vi "main.vi"() -> ()   [LabVIEW 2018]
uses:
  <vilib>/Platform/TimedLoop/XDataNode/timing_clust.ctl
  <vilib>/Platform/TimedLoop/XDataNode/nitl_modes.ctl
  <vilib>/Platform/TimedLoop/XDataNode/wakeup.ctl
  a5fe1e67-a595-4ba8-95b3-b389166d0479.vi
  fafd1210-cecf-4ec7-9a0a-c581520fbfe6.vi
  42531a82-c600-4602-b648-2c62e518af83.vi
  <vilib>/express/express shared/transition.llb/Dynamic To Waveform Array.vi
  <vilib>/express/express signal manip/GetorSetDDTAttributes/Set DDT Attributes/SetT0.vi
  <vilib>/express/express signal manip/GetorSetDDTAttributes/Set DDT Attributes/sub Set StartTimeStamp.vi
  <vilib>/express/express shared/transition.llb/Waveform Array To Dynamic.vi
  <vilib>/platform/TimedLoop/XDataNode/XDataNode.xnode
  <vilib>/express/express signal manip/GetorSetDDTAttributes/Set DDT Attributes/Set DDT Properties.xnode
  <vilib>/Platform/TimedLoop/XDataNode/XDNodeRunTimeDep.lvlib
  <vilib>/express/express signal manip/GetorSetDDTAttributes/Set DDT Attributes/Set DDT Attributes.lvlib
panel:
  in  "New file":bool
  out "Pending":i32
  out "RecordStatus":bool
  out "System State":T1(ring)
  in  "Overdrive":bool
  in  "Pause DAQ":bool
  in  "Record":bool
  in  "Log Folder":path=path "C:/LPLDocs"
  in  "Sensor Log Name":string="Log_Sensors"
  in  "Load Cell Log Name":string="Log_LoadCell"
  in  "Valve Log Name":string="Log_Valves"
  in  "Fire Sequence Tabs":T2(tab)
  in  "NC-F\nTiming":cluster{dbl, dbl, dbl, dbl, dbl, dbl}(slide)={0.0, 8.07, 10.0, 13.0, 13.0, 13.012830257415771} scale=0.0..13.0
  in  "NC-O\nTiming":cluster{dbl, dbl, dbl, dbl, dbl, dbl}(slide)={0.0, 8.05, 9.3, 13.0, 13.0, 13.012830257415771} scale=0.0..13.0
  in  "Ignitor\nTiming":cluster{dbl, dbl, dbl, dbl, dbl, dbl}(slide)={0.0, 9.8, 9.8, 13.0, 13.0, 13.012830257415771} scale=0.0..13.0
  in  "NC-FI\nTiming":cluster{dbl, dbl, dbl, dbl, dbl, dbl}(slide)={0.0, 15.0, 15.0, 15.0, 15.0, 0.0} scale=0.0..13.0
  in  "NC-OI\nTiming":cluster{dbl, dbl, dbl, dbl, dbl, dbl}(slide)={0.0, 15.0, 15.0, 15.0, 15.0, 0.0} scale=0.0..13.0
  in  "Fire\nTiming":cluster{dbl, dbl, dbl}(slide)={0.0, 10.0, 0.0} scale=0.0..13.0
  in  "NC-F Invert":bool
  in  "NC-O Invert":bool
  in  "Ignitor Invert":bool
  in  "NC-FI Invert":bool
  in  "NC-OI Invert":bool
  in  "ABORTED\nState":bool[](array[boolean])=[TRUE, TRUE, FALSE, FALSE, FALSE, FALSE]
  out "ABORTED Indicator":bool
  in  "Ignition Type":u16(ring)=2 items=["Spark Plug", "Glow Plug", "Pyrotechnic"]
  in  "Countdown + Fring\nLength":dbl=13.0
  in  "NC-F Open Delay":dbl=1.93
  in  "NC-O Open Delay":dbl=1.25
  in  "NC-FI Open Delay":dbl
  in  "Igniter Active Delay":dbl=1.0
  in  "NC-OI Open Delay":dbl
  in  "NC-F Close Delay":dbl
  in  "NC-O Close Delay":dbl
  in  "NC-FI Close Delay":dbl
  in  "Igniter Inactive Delay":dbl
  in  "NC-OI Close Delay":dbl
  in  "Edit Fire \nSequence":bool
  in  "SAFE State":bool[](array[boolean])=[FALSE, FALSE, FALSE, FALSE, FALSE, FALSE]
  in  "ARMED State":bool[](array[boolean])=[FALSE, TRUE, FALSE, FALSE, FALSE, FALSE]
  in  "Pressurized\nState":bool[](array[boolean])=[TRUE, TRUE, FALSE, FALSE, FALSE, FALSE]
  in  "Post-Fire\nState":bool[](array[boolean])=[TRUE, TRUE, FALSE, FALSE, FALSE, FALSE]
  out "Post-Fire Indicator":bool
  out "Pressurized Indicator":bool
  out "ARMED Indicator":bool
  out "SAFE Indicator":bool
  in  "Sensor Display":enum32{"Sensor Readouts", "Warning Limits"}(tab)
  out "PT-1P":dbl
  out "PT-2O":dbl
  out "PT-2P":dbl
  out "PT-3P":dbl
  out "PT-1F":dbl
  out "PT-1O":dbl
  out "PT-3E":dbl
  out "PT-2E":dbl
  out "PT-1E":dbl
  out "PT-CI":dbl
  out "PT-OI":dbl
  out "PT-FI":dbl
  out "PT-L":dbl
  out "TC-1P":dbl
  out "TC-2P":dbl
  out "TC-3P":dbl
  out "TC-1F":dbl
  out "TC-1O":dbl
  out "TC-2O":dbl
  out "FM-O":dbl
  out "LC-E":dbl
  out "FM-F":dbl
  in  "Error 4":dbl[](array[numeric])=[51.0, 31.0, 3500.0]
  in  "Error 1":dbl[](array[numeric])=[3500.0, 1700.0, 1700.0, 1700.0, 3500.0, 1700.0]
  in  "Warning 1":dbl[](array[numeric])=[2950.0, 1300.0, 1300.0, 1300.0, 2950.0, 1100.0]
  in  "Warning 2":dbl[](array[numeric])=[1300.0, 1100.0, 1300.0, 900.0, 900.0, 900.0, 100.0]
  in  "Error 2":dbl[](array[numeric])=[1700.0, 1700.0, 1700.0, 2500.0, 2500.0, 2500.0, 200.0]
  in  "Warning 3":dbl[](array[numeric])=[120.0, 120.0, 120.0, 120.0, 120.0, 120.0]
  in  "Error 3":dbl[](array[numeric])=[5000.0, 5000.0, 5000.0, 5000.0, 5000.0, 5000.0]
  in  "Warning 4":dbl[](array[numeric])=[45.0, 25.0, 2000.0]
  in  "Controls Tabs":enum32{"Manual Operations", "Fire Operations"}(tab)
  in  "NC-P":bool
  out "NC-P Status":bool
  in  "Actuate":bool
  in  "NO-P":bool
  out "NO-P Status":bool
  in  "NC-F":bool
  out "NC-F Status":bool
  in  "NC-FI":bool
  out "NC-FI Status":bool
  in  "NC-FP":bool
  out "NC-FP Status":bool
  in  "NC-O":bool
  out "NC-O Status":bool
  in  "NC-OI":bool
  out "NC-OI Status":bool
  in  "NC-OP":bool
  out "NC-OP Status":bool
  in  "Safety":bool
  in  "Ignition\nTest":bool
  in  "Pump":bool
  out "Fill Timer":dbl
  in  "Reset Timer":bool
  out "Fill Progress":dbl(slide) max=10.0 scale=0.0..50.0
  in  "Time Target":dbl=20.0
  in  "Ignition Type (Testing)":u16(ring)=2 items=["Spark Plug", "Glow Plug", "Pyrotechnic"]
  in  "Ignition ARM (Testing)":bool
  in  "Fire Button":bool
  in  "Abort Button":bool
  in  "Final Pre-fire Checklist":bool[](array[boolean])
  in  "ARM":bool
  out "ARM Indicator":bool
  in  "Pressurize":bool
  out "Pressurize Indicator":bool
  out "Countdown":dbl
  out "ERROR":bool
  # "Set file names \nBEFORE running!"
  # "Invert"
  # "Start"
  # "End"
  # "Countdown\nLength"
  # "Fire State"
  # "NC-P"
  # "Hardware Delays"
  # "Opening"
  # "Closing"
  # "NO-P"
  # "NC-F"
  # "NC-O"
  # "NC-F"
  # "Igniter"
  # "NC-FI"
  # "NC-FI"
  # "NC-OI"
  # "NC-O"
  # "NC-OI"
  # "TC-1P"
  # "f"
  # "PT-1P"
  # "psi"
  # "TC-2P"
  # "f"
  # "PT-2P"
  # "psi"
  # "TC-3P"
  # "f"
  # "PT-3P"
  # "psi"
  # "TC-1F"
  # "f"
  # "PT-1F"
  # "psi"
  # "TC-1O"
  # "f"
  # "PT-1O"
  # "psi"
  # "TC-2O"
  # "f"
  # "PT-2O"
  # "psi"
  # "PT-FI"
  # "psi"
  # "FM-F"
  # "gpm"
  # "PT-OI"
  # "psi"
  # "FM-O"
  # "acfm"
  # "PT-CI"
  # "psi"
  # "LC-E"
  # "lbf"
  # "psi"
  # "PT-1E"
  # "PT-2E"
  # "psi"
  # "PT-3E"
  # "psi"
  # "PT-L"
  # "psi"
  # "Warning\nThreshold"
  # "Error\nThreshold"
  # "Warning\nThreshold"
  # "Error\nThreshold"
  # "TC-1P"
  # "PT-1P"
  # "TC-2P"
  # "PT-2P"
  # "TC-3P"
  # "PT-3P"
  # "TC-1F"
  # "PT-1F"
  # "TC-2F"
  # "PT-1O"
  # "TC-3F"
  # "PT-2O"
  # "PT-FI"
  # "FM-F"
  # "PT-OI"
  # "(H2O Mass)"
  # "PT-CI"
  # "(JetA Mass)"
  # "PT-1E"
  # "FM-O"
  # "PT-2E"
  # "(N2 Mass)"
  # "PT-3E"
  # "(O2 Mass)"
  # "PT-L"
  # "LC-E"
  # "Ignition\nTest"
  # "Verify BOTH PANELS\nof the firing sequence\nare correctly configured"
  # "Verify all sensor readings\nare within acceptable\noperating conditions"
  # "Verify PA system is\noperational and range\nadmin is notified"
  # "Verify range is clear"
  # "Go/No go"
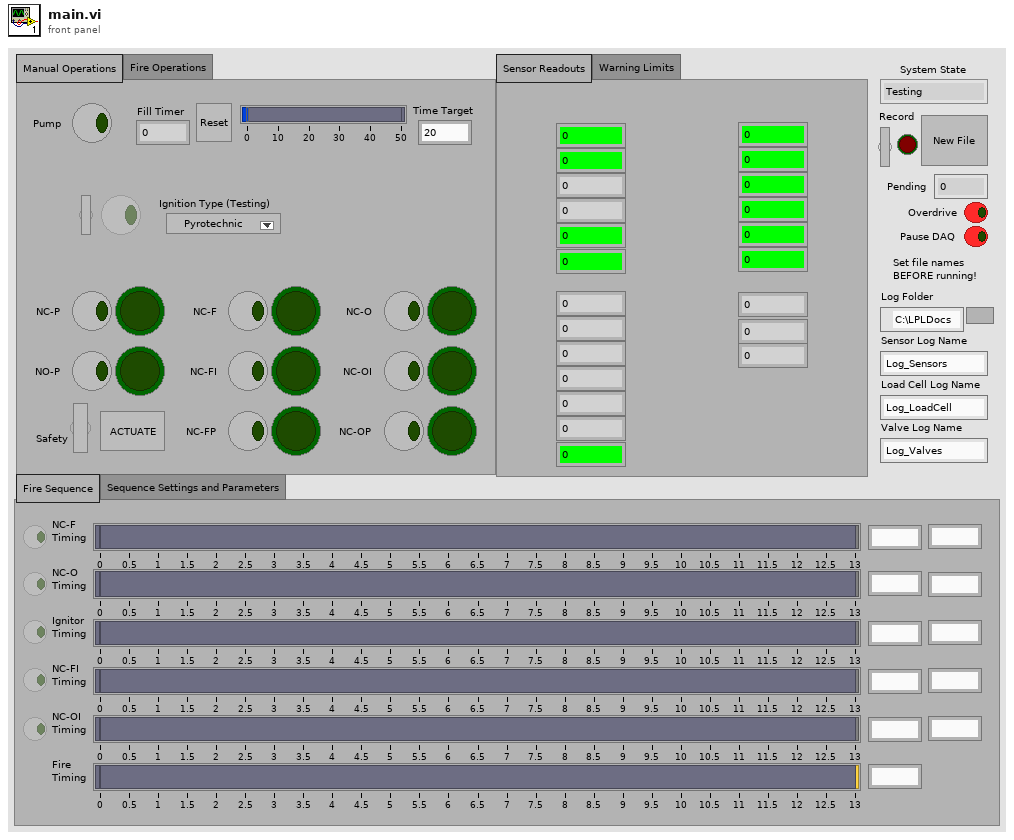
[diagram p1: front panel]
types:
  T1 = enum16{"Testing", "Safe", "Armed", "Pressurized", "Firing", "Aborted", "Fire Complete"}
  T2 = enum32{"Fire Sequence", "Sequence Settings and Parameters"}
  T3 = enum16{"Normal", "Overdrive", "Ready for Overdrive End", "Ready for new file", "New file"}
  T4 = cluster{"SensorPath":path, "LoadCellPath":path, "ValvePath":path}
  T5 = cluster{"LoadCell Queue":refnum<queue>, "Sensor Queue":refnum<queue>, "Valve Queue":refnum<queue>}
  T6 = cluster{"Sensors":refnum<notifier>, "LoadCell":refnum<notifier>, "Fileout":refnum<notifier>, "UI":refnum<notifier>}
  T7 = typedef "XDNodeRunTimeDep.lvlib/timing_clust.ctl" = cluster{"Expected End [f-1]":u64, "Actual End [f-1]":u64, "Finished Late? [f-1]":bool, "Expected End [i-1]":u64, "Actual End [i-1]":u64, "Finished Late? [i-1]":bool, "Expected Start [i]":u64, "Actual Start [i]":u64, "Expected Start [f]":u64, "Actual Start [f]":u64, "Source Name":string, "Structure Name":string, "Period":i64, "Deadline":i64, "Offset":i64, "Start":i64, "Priority":i32, "Timeout":i32, "Mode":T8, "Wakeup Reason":T9, "Error":errorcluster, "Source Type":string, "Secondary Source Type":string, "Global End Time":u64, "Global Start Time":u64, "Frame Duration":u64, "Iteration Duration":u64, "Assigned CPU":i32, "I/O Scan Engine Mode":u32}
  T8 = typedef "XDNodeRunTimeDep.lvlib/nitl_modes.ctl" = enum32{"No Change", "Process missed periods, maintain original phase", "Discard missed periods, maintain original phase", "Process missed periods, ignore original phase", "Discard missed periods, ignore original phase"}
  T9 = typedef "XDNodeRunTimeDep.lvlib/wakeup.ctl" = enum32{"Normal", "Aborted", "Asynchronous wakeup", "Timing source error", "Timed loop error", "Timeout"}
  T10 = enum16{"Default", "Record", "Overdrive", "Pause"}
  T11 = enum8{"Enabled", "Disabled", "Disabled and Grayed Out"}
  T12 = cluster{dbl, dbl, dbl, dbl, dbl, "Elapsed Time (s)":dbl}
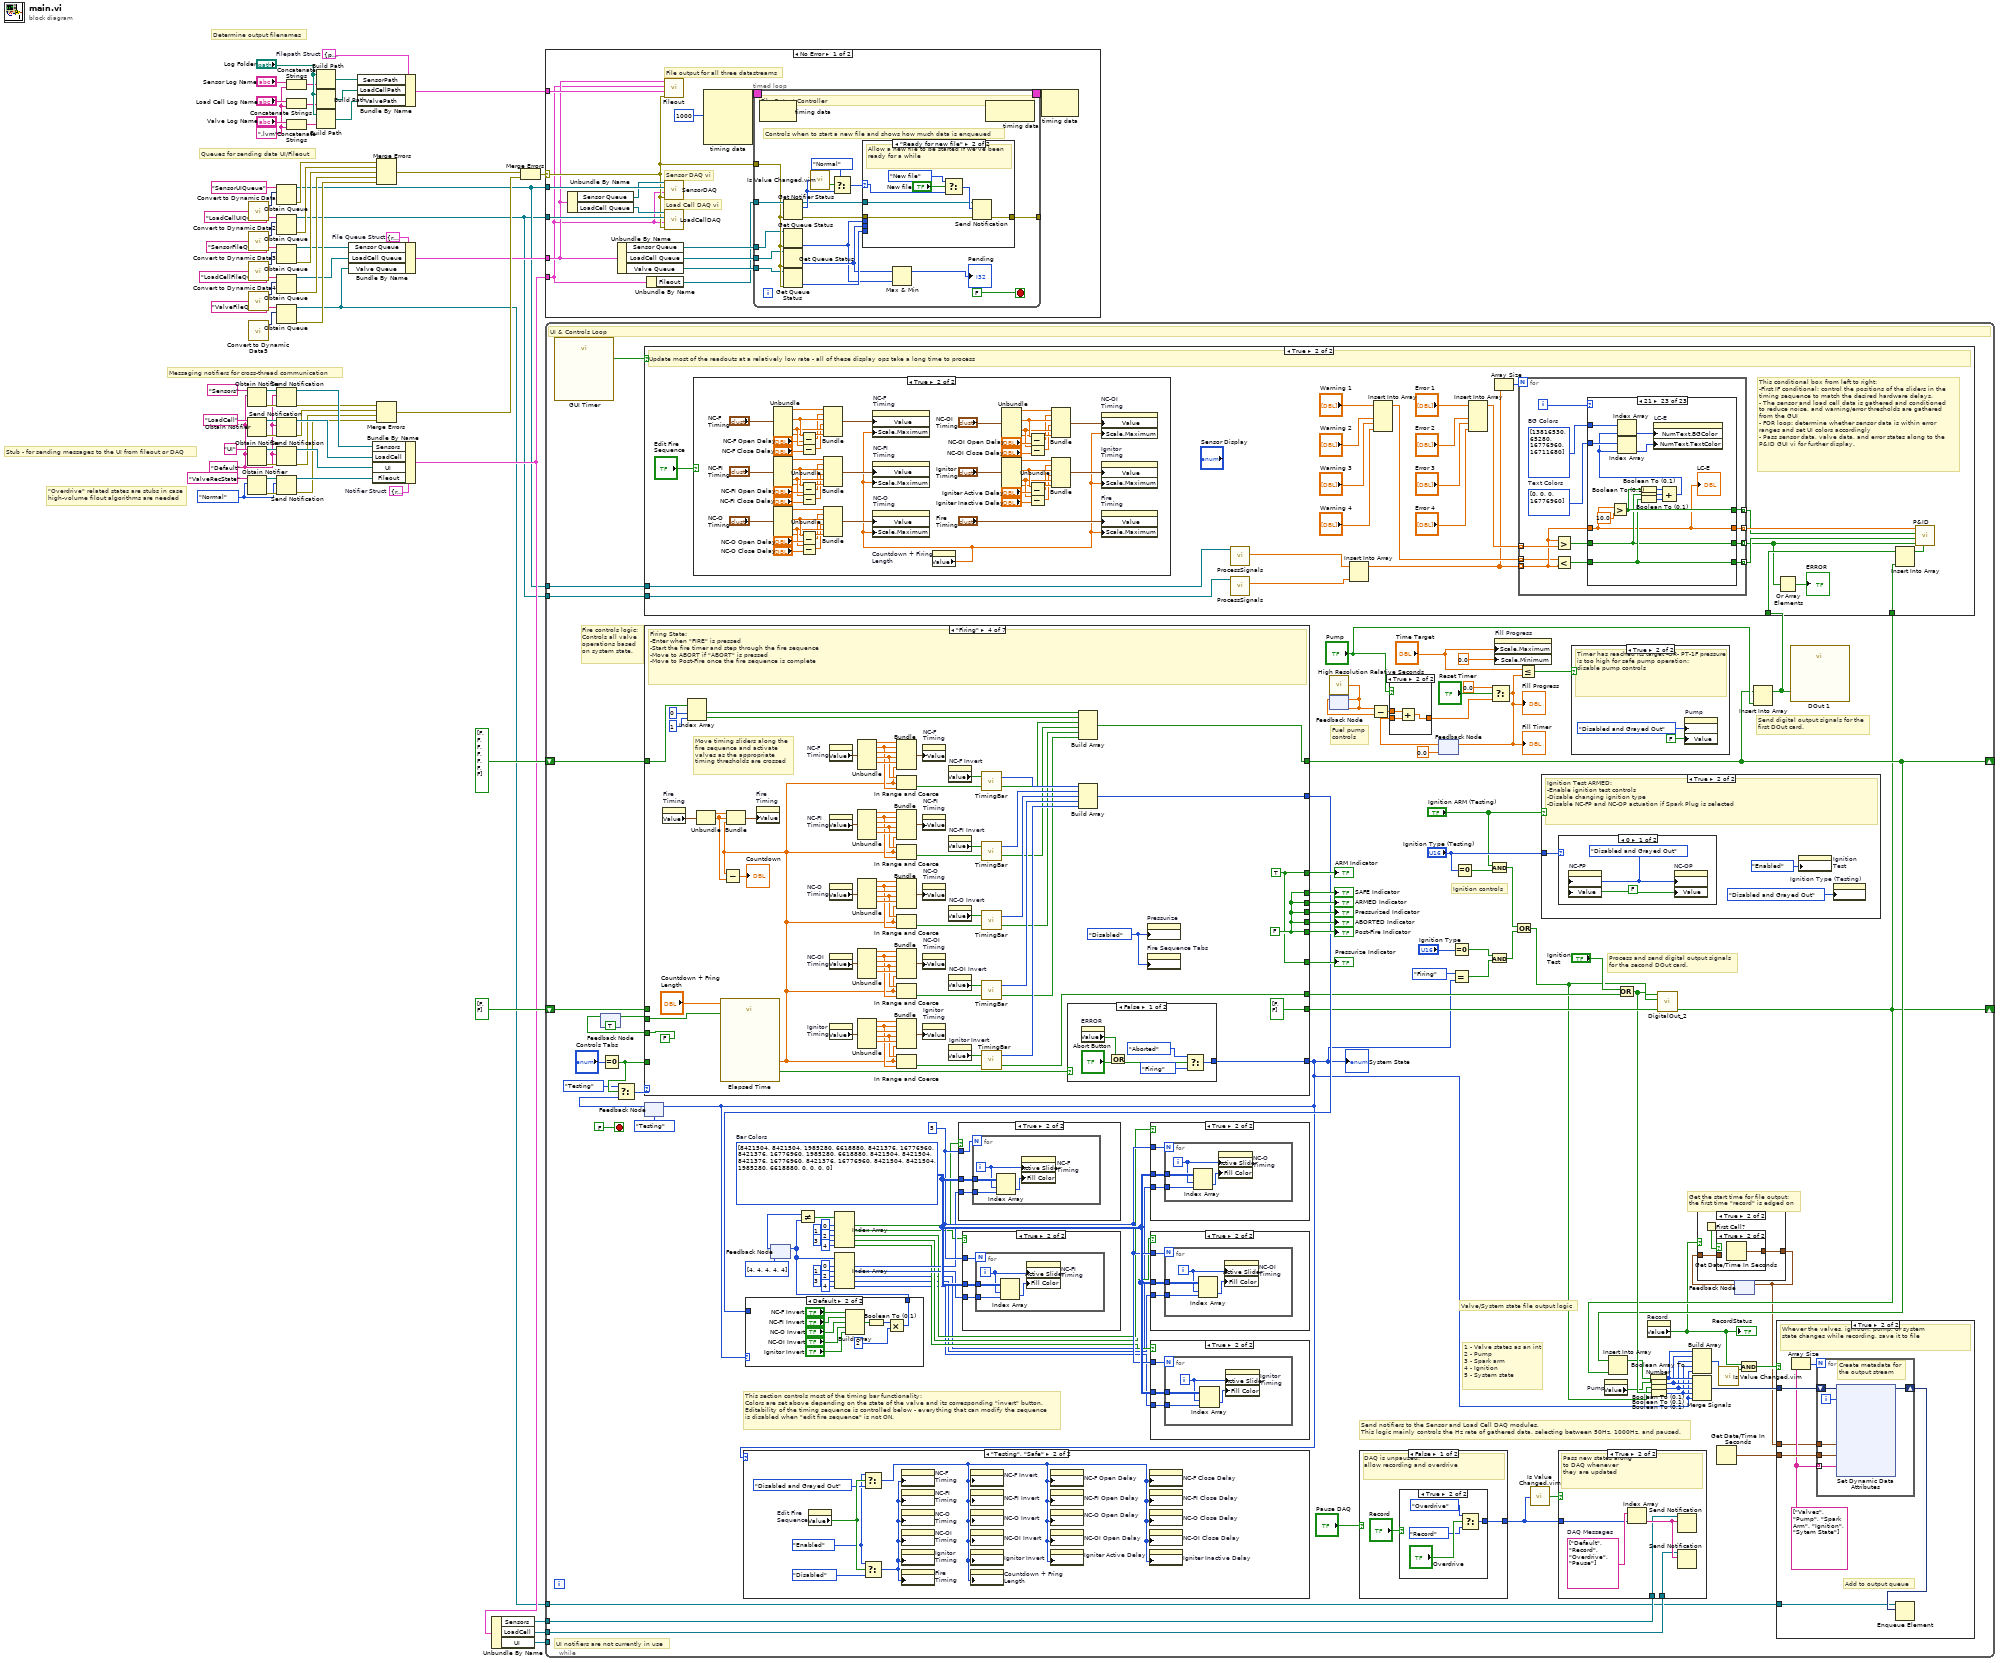
[diagram p0: block diagram]
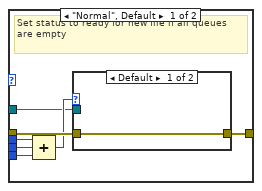
[diagram p2: hidden frame]
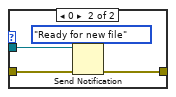
[diagram p3: hidden frame]
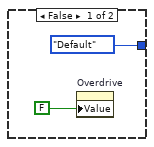
[diagram p9: hidden frame]
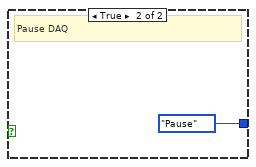
[diagram p10: hidden frame]
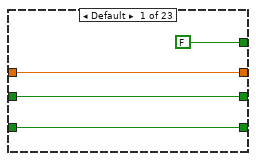
[diagram p13: hidden frame]
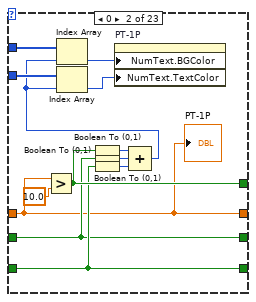
[diagram p14: hidden frame]
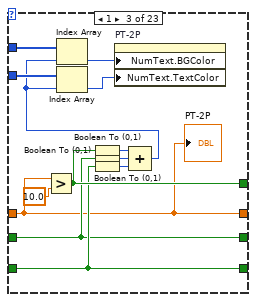
[diagram p15: hidden frame]
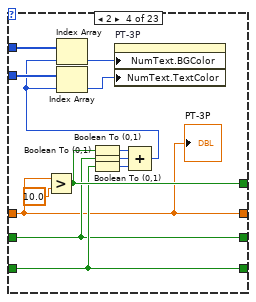
[diagram p16: hidden frame]
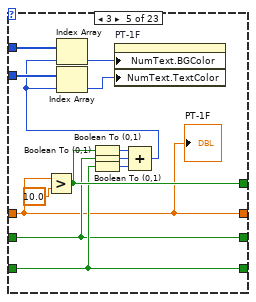
[diagram p17: hidden frame]
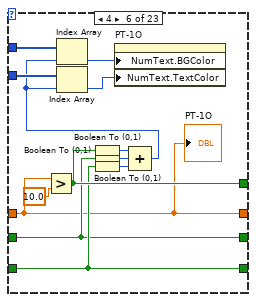
[diagram p18: hidden frame]
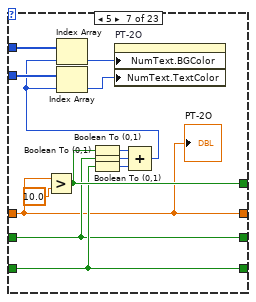
[diagram p19: hidden frame]
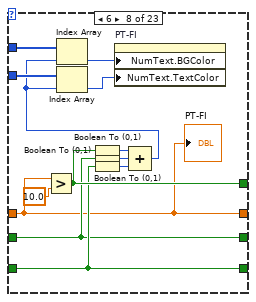
[diagram p20: hidden frame]
diagram:
  w13 = ".lvm"
  w21 = T3."Normal" ("RecState")
  w12 = T4 {"SensorPath"=path "", "LoadCellPath"=path "", "ValvePath"=path ""}  # Filepath Struct
  w8 = T5 {"LoadCell Queue"=refnum, "Sensor Queue"=refnum, "Valve Queue"=refnum}  # File Queue Struct
  w26 = T6 {"Sensors"=refnum, "LoadCell"=refnum, "Fileout"=refnum, "UI"=refnum}  # Notifier Struct
  w25 = "Default" ("RecState")
  # "Messaging notifiers for cross-thread communication"
  # "Queues for sending data UI/Fileout"
  # "Determine output filenames"
  # "Stub - for sending messages to the UI from fileout or DAQ"
  # "\"Overdrive\" related states are stubs in case\nhigh-volume filout algorithms are needed"
  n1 = Obtain Notifier(name (unnamed)="ValveRecState", notification data type=w21) -> (notifier out=w23:refnum<notifier>, error out=w22:errorcluster)  [unwired: 2 in, 1 out]
  n2 = Obtain Notifier(name (unnamed)="Sensors", notification data type=w25) -> (notifier out=w58:refnum<notifier>, error out=w57:errorcluster)  [unwired: 2 in, 1 out]
  n3 = Obtain Notifier(name (unnamed)="LoadCell", notification data type=w25) -> (notifier out=w60:refnum<notifier>, error out=w61:errorcluster)  [unwired: 2 in, 1 out]
  n4 = Obtain Notifier(name (unnamed)="UI", notification data type=w25) -> (notifier out=w62:refnum<notifier>, error out=w63:errorcluster)  [unwired: 2 in, 1 out]
  n5 = call "Convert to Dynamic Data"() -> ("Dynamic Data Type"=w47:dynamicdata)  [unwired: 4 in]
  n6 = call "Convert to Dynamic Data2"() -> ("Dynamic Data Type"=w45:dynamicdata)  [unwired: 4 in]
  n7 = call "Convert to Dynamic Data3"() -> ("Dynamic Data Type"=w43:dynamicdata)  [unwired: 4 in]
  n8 = call "Convert to Dynamic Data4"() -> ("Dynamic Data Type"=w41:dynamicdata)  [unwired: 4 in]
  n9 = call "Convert to Dynamic Data5"() -> ("Dynamic Data Type"=w39:dynamicdata)  [unwired: 4 in]
  n10 = Obtain Queue(name (unnamed)="SensorUIQueue", element data type=w47) -> (queue out=w2:refnum<queue>, error out=w38:errorcluster)  [unwired: 3 in, 1 out]
  n11 = Obtain Queue(name (unnamed)="LoadCellUIQueue", element data type=w45) -> (queue out=w1:refnum<queue>, error out=w37:errorcluster)  [unwired: 3 in, 1 out]
  n12 = Obtain Queue(name (unnamed)="SensorFileQueue", element data type=w43) -> (queue out=w7:refnum<queue>, error out=w36:errorcluster)  [unwired: 3 in, 1 out]
  n13 = Obtain Queue(name (unnamed)="LoadCellFileQueue", element data type=w41) -> (queue out=w6:refnum<queue>, error out=w35:errorcluster)  [unwired: 3 in, 1 out]
  n14 = Obtain Queue(name (unnamed)="ValveFileQueue", element data type=w39) -> (queue out=w5:refnum<queue>, error out=w34:errorcluster)  [unwired: 3 in, 1 out]
  n15 = Send Notification(notification=w25, notifier=w58, error in (no error)=w57) -> (notifier out=w55:refnum<notifier>, error out=w51:errorcluster)
  n16 = Send Notification(notification=w25, notifier=w60, error in (no error)=w61) -> (notifier out=w54:refnum<notifier>, error out=w50:errorcluster)
  n17 = Send Notification(notification=w25, notifier=w62, error in (no error)=w63) -> (notifier out=w53:refnum<notifier>, error out=w49:errorcluster)
  n18 = Send Notification(notification=w21, notifier=w23, error in (no error)=w22) -> (notifier out=w56:refnum<notifier>, error out=w52:errorcluster)
  n19 = Concatenate Strings("Sensor Log Name", w13) -> (w16:string)
  n20 = Concatenate Strings("Load Cell Log Name", w13) -> (w15:string)
  n21 = Concatenate Strings("Valve Log Name", w13) -> (w14:string)
  n22 = Build Path(base path="Log Folder", name or relative path=w16) -> (appended path=w11:path)
  n23 = Build Path(base path="Log Folder", name or relative path=w15) -> (appended path=w10:path)
  n24 = Build Path(base path="Log Folder", name or relative path=w14) -> (appended path=w9:path)
  n25 = Bundle By Name(cluster=w8, "Sensor Queue"=w7, "LoadCell Queue"=w6, "Valve Queue"=w5) -> (w4:T5)
  n26 = Bundle By Name(cluster=w12, "SensorPath"=w11, "LoadCellPath"=w10, "ValvePath"=w9) -> (w3:T4)
  n27 = Bundle By Name(cluster=w26, "Sensors"=w55, "LoadCell"=w54, "UI"=w53, "Fileout"=w56) -> (w33:T6)
  n28 = Merge Errors(w38, w37, w36, w35, w34) -> (w29:errorcluster)
  n29 = Merge Errors(w51, w50, w49, w52) -> (w28:errorcluster)
  n30 = Unbundle By Name(w33) -> ("Sensors"=w32:refnum<notifier>, "LoadCell"=w31:refnum<notifier>, "UI"=w30:refnum<notifier>)
  n31 = Merge Errors(w29, w28) -> (w27:errorcluster)
  n32 = case shown="No Error" w27 {
    selector: w27 -> [w75 _]
    tunnel: w33 -> [w72 _]
    tunnel: w4 -> [w73 _]
    tunnel: w3 -> [w82 _]
    tunnel: w2 -> [w81 _]
    tunnel: w1 -> [w80 _]
    frame No Error {
      # "File output for all three datastreams"
      # "Load Cell DAQ vi"
      # "Sensor DAQ vi"
      n33 = Unbundle By Name(w73) -> ("Sensor Queue"=w78:refnum<queue>, "LoadCell Queue"=w79:refnum<queue>)
      n34 = Unbundle By Name(w73) -> ("Sensor Queue"=w69:refnum<queue>, "LoadCell Queue"=w70:refnum<queue>, "Valve Queue"=w71:refnum<queue>)
      n35 = Unbundle By Name(w72) -> ("Fileout"=w68:refnum<notifier>)
      n36 = call "Fileout.vi"("error in (no error)"=w75, "Filepaths"=w82, "Message Notifiers"=w72, "File Queues"=w73) -> ()  [unwired: 7 in, 1 out]
      n37 = call "SensorDAQ.vi"("error in (no error)"=w75, "Message Notifiers"=w72, "UI Queue"=w81, "Logging Queue"=w78) -> ()  [unwired: 7 in, 1 out]
      n38 = call "LoadCellDAQ.vi"("error in (no error)"=w75, "Message Notifiers"=w72, "UI Queue"=w80, "Logging Queue"=w79) -> ()  [unwired: 7 in, 1 out]
      n39 = node-c288(i64 1000 ("Period")) -> (w77:T7)  [unwired: 3 in]
      n40 = timed-loop {
        tunnel: [w98] -> _
        tunnel: w68 -> [w93]
        tunnel: w75 -> [w90]
        timing: w77 -> [_]
        timing-out: [_] -> w76
        tunnel: w69 -> [w89]
        tunnel: w70 -> [w88]
        tunnel: w71 -> [w87]
        stop <- FALSE stop-if-true
        # "Controls when to start a new file and shows how much data is enqueued"
        # "File Output Controller"
        n41 = node-c288() -> ()  [unwired: 1 in, 1 out]
        n42 = Get Notifier Status(notifier=w93, error in (no error)=w90) -> (notifier out=w92:refnum<notifier>, current notification=w96:T3, error out=w97:errorcluster)  [unwired: 2 out]
        n43 = Get Queue Status(queue=w89, error in (no error)=w90) -> (# elements in queue=w84:i32)  [unwired: 1 in, 7 out]
        n44 = Get Queue Status(queue=w88, error in (no error)=w90) -> (# elements in queue=w85:i32)  [unwired: 1 in, 7 out]
        n45 = Get Queue Status(queue=w87, error in (no error)=w90) -> (# elements in queue=w86:i32)  [unwired: 1 in, 7 out]
        n46 = call "Is Value Changed.vim"("value"=w96) -> ("changed or first call?"=w95:bool)
        n47 = Select(t=T3."Normal" ("RecState"), s=w95, f=w96) -> (s? t:f=w91:T3)
        n48 = case shown="\"Ready for new file\"" w91 {
          selector: w91 -> [_ w120]
          tunnel: [w108 w117] -> w98
          tunnel: w97 -> [w107 w116]
          tunnel: w92 -> [w105 w115]
          tunnel: w84 -> [w104 _]
          tunnel: w85 -> [w103 _]
          tunnel: w86 -> [w102 _]
          frame "Normal", Default {
            # "Set status to ready for new file if all queues are empty"
            n49 = Compound Arithmetic op=ADD(w104, w103, w102) -> (w106:i32)
            n50 = case shown="Default" w106 {
              tunnel: [w109 w113] -> w108
              tunnel: w107 -> [w109 w112]
              tunnel: w105 -> [_ w110]
              frame Default {
              }
              frame 0 {
                n51 = Send Notification(notification=T3."Ready for new file" ("RecState"), notifier=w110, error in (no error)=w112) -> (error out=w113:errorcluster)  [unwired: 1 out]
              }
            }
          }
          frame "Ready for new file" {
            # "Allow a new file to be started if we've been ready for a while"
            n52 = Select(t=T3."New file" ("RecState"), s="New file", f=w120) -> (s? t:f=w118:T3)
            n53 = Send Notification(notification=w118, notifier=w115, error in (no error)=w116) -> (error out=w117:errorcluster)  [unwired: 1 out]
          }
        }
        n54 = Max & Min(x=w85, y=w84) -> (max(x,y)=→"Pending":i32)  [unwired: 1 out]
        n55 = node-c288() -> ()  [unwired: 1 in, 1 out]
      }
      n56 = node-c288(w76) -> ()  [unwired: 1 out]
    }
    frame Error {
    }
  }
  n57 = while {
    shift-right: [w143] -> _
    shift-left: bool[] [FALSE, FALSE, FALSE, FALSE, FALSE, FALSE, FALSE] -> [w204]
    shift-right: [w136] -> _
    shift-left: bool[] [FALSE, FALSE] -> [w205]
    tunnel: w2 -> [w152]
    tunnel: w1 -> [w151]
    tunnel: w32 -> [w146]
    tunnel: w31 -> [w145]
    tunnel: [w150] -> _
    tunnel: w30 -> [w150]
    tunnel: w5 -> [w142]
    stop <- FALSE stop-if-true
    w200 = 5
    w201 = u32[][] [[8421504, 8421504, 1985280, 6618880], [8421376, 16776960, 8421376, 16776960], [1985280, 6618880, 8421504, 8421504], [8421376, 16776960, 8421376, 16776960], [8421504, 8421504, 1985280, 6618880], [0, 0, 0, 0]]  # Bar Colors
    # "Get the start time for file output:\nthe first time \"record\" is edged on"
    # "1 - Valve states as an int\n2 - Pump\n3 - Spark arm\n4 - Ignition\n5 - System state"
    # "Valve/System state file output logic"
    # "UI notifiers are not currently in use"
    # "Fire controls logic:\nControls all valve\noperations based\non system state."
    # "Send notifiers to the Sensor and Load Cell DAQ modules.\nThis logic mainly controls the Hz rate of gathered data, selecting between 50Hz, 1000Hz, and paused."
    # "Ignition controls"
    # "Fuel pump\ncontrols"
    # "Send digital output signals for the\nfirst DOut card."
    # "Process and send digital output signals\nfor the second DOut card."
    # "This section controls most of the timing bar functionality:\nColors are set above depending on the state of the valve and its corresponding \"invert\" button.\nEditability of the timing sequence is controlled below - everything that can modify the sequence\nis disabled when \"edit fire sequence\" is not ON."
    # "UI & Controls Loop"
    n58 = call "GUI Timer"() -> ("Time has Elapsed"=w153:bool)  [unwired: 12 in, 7 out]
    n59 = feedback #1(TRUE) -> (w173:bool)
    n60 = Equal To 0?(x="Controls Tabs") -> (x = 0?=w208:bool)
    n61 = feedback #2(T1."Testing" ("System State")) -> (w175:T1)
    n62 = Select(t=T1."Testing" ("System State"), s=w208, f=w175) -> (s? t:f=w209:T1)
    n63 = case shown="\"Firing\"" w209 {
      tunnel: [w708 w723 w750 w827 w844 w850 w865] -> w211
      tunnel: [w708 w723 w750 w827 w840 w854 w865] -> w212
      tunnel: [w708 w723 w736 w827 w844 w854 w865] -> w207
      tunnel: [w708 w724 w750 w827 w844 w854 w865] -> w206
      tunnel: [TRUE w723 w750 w827 w844 w854 w865] -> w213
      tunnel: ["SAFE State" "ARMED State" "Pressurized\nState" w769 "ABORTED\nState" "Post-Fire\nState" w866] -> w143
      tunnel: [w713 w727 w740 w825 T1."Aborted" ("System State") T1."Fire Complete" ("System State") w907] -> w126
      tunnel: w208 -> [_ _ _ _ _ _ w904]
      tunnel: [bool[] [FALSE, FALSE] bool[] [FALSE, FALSE] bool[] [FALSE, FALSE] bool[] [FALSE, FALSE] bool[] [FALSE, FALSE] bool[] [FALSE, FALSE] w867] -> w163
      tunnel: w205 -> [_ _ _ _ _ _ w869]
      tunnel: w204 -> [_ _ _ w754 _ _ w868]
      tunnel: [w708 w724 w736 w823 w840 w850 w865] -> w203
      tunnel: [w708 w723 w736 w823 w840 w850 w865] -> w202
      tunnel: [i32[] [0, 0, 0, 0, 0] i32[] [0, 0, 0, 0, 0] i32[] [0, 0, 0, 0, 0] w812 i32[] [0, 0, 0, 0, 0] i32[] [0, 0, 0, 0, 0] i32[] [0, 0, 0, 0, 0]] -> w171
      tunnel: [TRUE TRUE TRUE FALSE FALSE FALSE TRUE] -> w174
      tunnel: w173 -> [_ _ _ w757 _ _ _]
      tunnel: [FALSE ("Valve Status") FALSE ("Valve Status") FALSE ("Valve Status") w751 FALSE ("Valve Status") FALSE ("Valve Status") FALSE ("Valve Status")] -> w162
      frame "Safe" {
        w708 = FALSE
        # "SAFE State:\n-Enter when \"Firing Operations\" tab is selected\n-Move to ARMED when \"ARM\" is switched on"
        n64 = property on="Pump" class="Bool (strict)"("Value"=FALSE ("Pump")) -> ()  [unwired: 2 in, 2 out]
        n65 = property on="Ignition\nTest" class="Bool (strict)"("Value"=FALSE ("Ignition\nTest")) -> ()  [unwired: 2 in, 2 out]
        n66 = property on="Edit Fire \nSequence" class="Bool (strict)"("DisabledEnum"=T11."Disabled and Grayed Out" ("Disabled"), "Value"=FALSE ("Edit Fire \nSequence")) -> ()  [unwired: 2 in, 2 out]
        n67 = Select(t=T1."Armed" ("System State"), s="ARM", f=T1."Safe" ("System State")) -> (s? t:f=w713:T1)
      }
      frame "Armed" {
        w724 = TRUE
        w723 = FALSE
        # "ARMED State:\n-Enter when \"ARM\" is switched on\n-Move to Pressurized when \"Pressurize\" is switched on"
        n68 = property on="ARM" class="Bool (strict)"("DisabledEnum"=T11."Disabled" ("Disabled")) -> ()  [unwired: 2 in, 2 out]
        n69 = property on="Pressurize" class="Bool (strict)"("DisabledEnum"=T11."Enabled" ("Disabled")) -> ()  [unwired: 2 in, 2 out]
        n70 = Select(t=T1."Pressurized" ("System State"), s="Pressurize", f=T1."Armed" ("System State")) -> (s? t:f=w727:T1)
      }
      frame "Pressurized" {
        w750 = FALSE
        w736 = TRUE
        # "Pressurized State\n-Enter when \"Pressurize\" is switched on\n-Move to Firing when the pre-fire checklist is complete and \"FIRE\" is pressed"
        n71 = Equal To 0?(x="Fire Sequence Tabs") -> (x = 0?=w746:bool)
        n72 = Build Array (concatenate)("Final Pre-fire Checklist", w746) -> (w745:bool[])
        n73 = And Array Elements(Boolean array=w745) -> (logical AND=w744:bool)
        n74 = Select(t=T11."Enabled" ("Disabled"), s=w744, f=T11."Disabled and Grayed Out" ("Disabled")) -> (s? t:f=w743:T11)
        n75 = property on="Pressurize" class="Bool (strict)"("DisabledEnum"=T11."Disabled" ("Disabled")) -> ()  [unwired: 2 in, 2 out]
        n76 = property on="Fire Button" class="Bool"("DisabledEnum"=w743) -> ()  [unwired: 2 in, 2 out]
        n77 = Select(t=T1."Firing" ("System State"), s="Fire Button", f=T1."Pressurized" ("System State")) -> (s? t:f=w740:T1)
      }
      frame "Firing" {
        w823 = TRUE
        w826 = T11."Disabled" ("Disabled")
        w827 = FALSE
        # "Move timing sliders along the\nfire sequence and activate\nvalves as the appropriate\ntiming thresholds are crossed"
        # "Firing State:\n-Enter when \"FIRE\" is pressed\n-Start the fire timer and step through the fire sequence\n-Move to ABORT if \"ABORT\" is pressed\n-Move to Post-Fire once the fire sequence is complete"
        n78 = property on="Fire\nTiming" class="Slide (strict)"() -> ("Value"=w764:cluster{dbl, dbl, dbl})  [unwired: 2 in, 2 out]
        n79 = Index Array(array=w754, index #1=0 ("index"), index #2=1 ("index")) -> (element #1=w753:bool, element #2=w752:bool)
        n80 = Unbundle(w764) -> (w763:dbl, w760:dbl)  [unwired: 1 out]
        n81 = call "Elapsed Time"("Time Target (s)"="Countdown + Fring\nLength", "Reset"=w757) -> ("Elapsed Time (s)"=w761:dbl, "Time has Elapsed"=w813:bool)  [unwired: 10 in, 6 out]
        n82 = Subtract(x=w761, y=w760) -> (x-y=→"Countdown":dbl)
        n83 = Bundle(w763, w760, "Elapsed Time (s)"=w761) -> (w762:cluster{dbl, dbl, "Elapsed Time (s)":dbl})  [unwired: 1 in]
        n84 = property on="Fire\nTiming" class="Slide (strict)"("Value"=w762) -> ()  [unwired: 2 in, 2 out]
        n85 = property on="NC-F\nTiming" class="Slide (strict)"() -> ("Value"=w810:cluster{dbl, dbl, dbl, dbl, dbl, dbl})  [unwired: 2 in, 2 out]
        n86 = property on="NC-FI\nTiming" class="Slide (strict)"() -> ("Value"=w783:cluster{dbl, dbl, dbl, dbl, dbl, dbl})  [unwired: 2 in, 2 out]
        n87 = property on="NC-O\nTiming" class="Slide (strict)"() -> ("Value"=w801:cluster{dbl, dbl, dbl, dbl, dbl, dbl})  [unwired: 2 in, 2 out]
        n88 = property on="NC-OI\nTiming" class="Slide (strict)"() -> ("Value"=w792:cluster{dbl, dbl, dbl, dbl, dbl, dbl})  [unwired: 2 in, 2 out]
        n89 = property on="Ignitor\nTiming" class="Slide (strict)"() -> ("Value"=w822:cluster{dbl, dbl, dbl, dbl, dbl, dbl})  [unwired: 2 in, 2 out]
        n90 = Unbundle(w810) -> (w807:dbl, w805:dbl, w809:dbl, w806:dbl, w808:dbl)  [unwired: 1 out]
        n91 = Unbundle(w783) -> (w780:dbl, w778:dbl, w782:dbl, w779:dbl, w781:dbl)  [unwired: 1 out]
        n92 = Unbundle(w801) -> (w798:dbl, w796:dbl, w800:dbl, w797:dbl, w799:dbl)  [unwired: 1 out]
        n93 = Unbundle(w792) -> (w789:dbl, w787:dbl, w791:dbl, w788:dbl, w790:dbl)  [unwired: 1 out]
        n94 = Unbundle(w822) -> (w819:dbl, w817:dbl, w821:dbl, w818:dbl, w820:dbl)  [unwired: 1 out]
        n95 = Bundle(w807, w805, w809, w806, w808, "Elapsed Time (s)"=w761) -> (w802:T12)  [unwired: 1 in]
        n96 = In Range and Coerce(upper limit=w806, x=w761, lower limit=w805) -> (In Range?=w804:bool)  [unwired: 1 out]
        n97 = Bundle(w780, w778, w782, w779, w781, "Elapsed Time (s)"=w761) -> (w775:T12)  [unwired: 1 in]
        n98 = In Range and Coerce(upper limit=w779, x=w761, lower limit=w778) -> (In Range?=w777:bool)  [unwired: 1 out]
        n99 = Bundle(w798, w796, w800, w797, w799, "Elapsed Time (s)"=w761) -> (w793:T12)  [unwired: 1 in]
        n100 = In Range and Coerce(upper limit=w797, x=w761, lower limit=w796) -> (In Range?=w795:bool)  [unwired: 1 out]
        n101 = Bundle(w789, w787, w791, w788, w790, "Elapsed Time (s)"=w761) -> (w784:T12)  [unwired: 1 in]
        n102 = In Range and Coerce(upper limit=w788, x=w761, lower limit=w787) -> (In Range?=w786:bool)  [unwired: 1 out]
        n103 = Bundle(w819, w817, w821, w818, w820, "Elapsed Time (s)"=w761) -> (w811:T12)  [unwired: 1 in]
        n104 = In Range and Coerce(upper limit=w818, x=w761, lower limit=w817) -> (In Range?=w815:bool)  [unwired: 1 out]
        n105 = property on="NC-F\nTiming" class="Slide (strict)"("Value"=w802) -> ()  [unwired: 2 in, 2 out]
        n106 = property on="NC-FI\nTiming" class="Slide (strict)"("Value"=w775) -> ()  [unwired: 2 in, 2 out]
        n107 = property on="NC-O\nTiming" class="Slide (strict)"("Value"=w793) -> ()  [unwired: 2 in, 2 out]
        n108 = property on="NC-OI\nTiming" class="Slide (strict)"("Value"=w784) -> ()  [unwired: 2 in, 2 out]
        n109 = property on="Ignitor\nTiming" class="Slide (strict)"("Value"=w811) -> ()  [unwired: 2 in, 2 out]
        n110 = property on="NC-F Invert" class="Bool (strict)"() -> ("Value"=w803:bool)  [unwired: 2 in, 2 out]
        n111 = property on="NC-FI Invert" class="Bool (strict)"() -> ("Value"=w776:bool)  [unwired: 2 in, 2 out]
        n112 = property on="NC-O Invert" class="Bool (strict)"() -> ("Value"=w794:bool)  [unwired: 2 in, 2 out]
        n113 = property on="NC-OI Invert" class="Bool (strict)"() -> ("Value"=w785:bool)  [unwired: 2 in, 2 out]
        n114 = property on="Ignitor Invert" class="Bool (strict)"() -> ("Value"=w814:bool)  [unwired: 2 in, 2 out]
        n115 = call "TimingBar.vi"("Timer Within Range"=w804, "Inverted"=w803) -> ("Valve Status"=w768:bool, "Color Index"=w774:i32)
        n116 = call "TimingBar.vi"("Timer Within Range"=w777, "Inverted"=w776) -> ("Valve Status"=w767:bool, "Color Index"=w773:i32)
        n117 = call "TimingBar.vi"("Timer Within Range"=w795, "Inverted"=w794) -> ("Valve Status"=w766:bool, "Color Index"=w772:i32)
        n118 = call "TimingBar.vi"("Timer Within Range"=w786, "Inverted"=w785) -> ("Valve Status"=w765:bool, "Color Index"=w771:i32)
        n119 = call "TimingBar.vi"("Timer Within Range"=w815, "Inverted"=w814) -> ("Valve Status"=w751:bool, "Color Index"=w770:i32)
        n120 = case shown="False" w813 {
          tunnel: [w833 T1."Fire Complete" ("System State")] -> w825
          frame False {
            n121 = property on="ERROR" class="Bool (strict)"() -> ("Value"=w828:bool)  [unwired: 2 in, 2 out]
            n122 = Or(x=w828, y="Abort Button") -> (x .or. y?=w829:bool)
            n123 = Select(t=T1."Aborted" ("System State"), s=w829, f=T1."Firing" ("System State")) -> (s? t:f=w833:T1)
          }
          frame True {
          }
        }
        n124 = Build Array(w753, w752, w768, w767, w766, w765) -> (w769:bool[])
        n125 = Build Array(w774, w773, w772, w771, w770) -> (w812:i32[])
        n126 = property on="Pressurize" class="Bool (strict)"("DisabledEnum"=w826) -> ()  [unwired: 2 in, 2 out]
        n127 = property on="Fire Sequence Tabs" class="TabCtl (strict)"("DisabledEnum"=w826) -> ()  [unwired: 2 in, 2 out]
      }
      frame "Aborted" {
        w840 = TRUE
        w844 = FALSE
        # "ABORTED State:\n-Enter when \"ABORT\" is pressed\n-Stay here until the Manual Operations tab is selected (goes to Testing State)"
        n128 = property on="Fire Sequence Tabs" class="TabCtl (strict)"("DisabledEnum"=T11."Enabled" ("Disabled")) -> ()  [unwired: 2 in, 2 out]
        n129 = property on="Fire Button" class="Bool"("DisabledEnum"=T11."Disabled and Grayed Out" ("Disabled")) -> ()  [unwired: 2 in, 2 out]
      }
      frame "Fire Complete" {
        w854 = FALSE
        w850 = TRUE
        # "Post Fire State:\n-Enter when the Fire sequence is completed\n-Stay here until the Manual Operations tab is selected (goes to Testing State)"
        n130 = property on="Fire Button" class="Bool"("DisabledEnum"=T11."Disabled and Grayed Out" ("Disabled")) -> ()  [unwired: 2 in, 2 out]
        n131 = property on="Fire Sequence Tabs" class="TabCtl (strict)"("DisabledEnum"=T11."Enabled" ("Disabled")) -> ()  [unwired: 2 in, 2 out]
      }
      frame "Testing", Default {
        w905 = T11."Disabled and Grayed Out" ("Disabled")
        w906 = FALSE ("ARM")
        w908 = T11."Enabled" ("Disabled")
        w865 = FALSE
        # "Testing State:\n-Enter whenever the Manual Operations tab is selected\n-Allow manual actuation of all valves\n-Ignition system testing\n-Fuel Pump operation"
        n132 = property on="Fire\nTiming" class="Slide (strict)"() -> ("Value"=w862:cluster{dbl, dbl, dbl})  [unwired: 2 in, 2 out]
        n133 = Build Array("NC-P", "NO-P", "NC-F", "NC-FI", "NC-O", "NC-OI") -> (w870:bool[])
        n134 = Unbundle(w862) -> (w861:dbl)  [unwired: 2 out]
        n135 = And(x=w870, y="Actuate") -> (x .and. y?=w881:bool[])
        n136 = Subtract(x=0.0, y=w861) -> (x-y=w859:dbl)
        n137 = Exclusive Or(1:w881, 2:w868) -> (0:w866:bool[])
        n138 = property on="Countdown" class="DigNum (strict)"("Value"=w859) -> ()  [unwired: 2 in, 2 out]
        n139 = Build Array("NC-FP", "NC-OP") -> (w879:bool[])
        n140 = And(x=w879, y="Actuate") -> (x .and. y?=w882:bool[])
        n141 = Exclusive Or(1:w869, 2:w882) -> (0:w867:bool[])
        n142 = property on="Ignition Type (Testing)" class="Ring (strict)"() -> ("Value"=w887:u16)  [unwired: 2 in, 2 out]
        n143 = Equal To 0?(x=w887) -> (x = 0?=w889:bool)
        n144 = Or Array Elements(Boolean array=w867) -> (logical OR=w888:bool)
        n145 = Index Array(array=w867, index #1=0 ("index"), index #2=1 ("index")) -> (element #1=→"NC-FP Status":bool, element #2=→"NC-OP Status":bool)
        n146 = And(x=w889, y=w888) -> (x .and. y?=w890:bool)
        n147 = Index Array(array=w866, index #1=0 ("index"), index #2=1 ("index"), index #3=2 ("index"), index #4=3 ("index"), index #5=4 ("index"), index #6=5 ("index")) -> (element #1=→"NC-P Status":bool, element #2=→"NO-P Status":bool, element #3=→"NC-F Status":bool, element #4=→"NC-FI Status":bool, element #5=→"NC-O Status":bool, element #6=→"NC-OI Status":bool)
        n148 = case shown="False" "Safety" {
          frame False {
            # "Actuation SAFE:\n-Disable actuation"
            n149 = property on="Actuate" class="Bool"("DisabledEnum"=T11."Disabled and Grayed Out" ("Disabled")) -> ()  [unwired: 2 in, 2 out]
          }
          frame True {
            # "Actuation ARMED:\n-Enable Actiuation"
            n150 = property on="Actuate" class="Bool"("DisabledEnum"=T11."Enabled" ("Disabled")) -> ()  [unwired: 2 in, 2 out]
          }
        }
        n151 = case shown="True" w890 {
          frame False {
            # "Purge Valves closed:\n-Allow Ignition Test ARM"
            n152 = property on="Ignition ARM (Testing)" class="Bool (strict)"("DisabledEnum"=T11."Enabled" ("Disabled")) -> ()  [unwired: 2 in, 2 out]
          }
          frame True {
            # "Any Purge valve open AND Spark Plug selected:\n-Disable Ignition ARM"
            n153 = property on="Ignition ARM (Testing)" class="Bool (strict)"("DisabledEnum"=T11."Disabled and Grayed Out" ("Disabled")) -> ()  [unwired: 2 in, 2 out]
          }
        }
        n154 = property on="Final Pre-fire Checklist" class="Arr (strict)"("Value"=bool[] [FALSE, FALSE, FALSE, FALSE, FALSE]) -> ()  [unwired: 2 in, 2 out]
        n155 = property on="Edit Fire \nSequence" class="Bool (strict)"("DisabledEnum"=w908) -> ()  [unwired: 2 in, 2 out]
        n156 = property on="ARM" class="Bool (strict)"("DisabledEnum"=w908, "Value"=w906) -> ()  [unwired: 2 in, 2 out]
        n157 = property on="Pressurize" class="Bool (strict)"("DisabledEnum"=w905, "Value"=w906) -> ()  [unwired: 2 in, 2 out]
        n158 = property on="Fire Button" class="Bool"("DisabledEnum"=w905) -> ()  [unwired: 2 in, 2 out]
        n159 = Select(t=T1."Testing" ("System State"), s=w904, f=T1."Safe" ("System State")) -> (s? t:f=w907:T1)
      }
    }
    "Post-Fire Indicator" <- w211
    "Pressurized Indicator" <- w207
    "ARMED Indicator" <- w206
    "ABORTED Indicator" <- w212
    "SAFE Indicator" <- w213
    "ARM Indicator" <- w203
    "Pressurize Indicator" <- w202
    "System State" <- w126
    n160 = feedback-in #1(w174) -> ()
    n161 = feedback-in #2(w126) -> ()
    n162 = case shown="\"Testing\", \"Safe\"" w126 {
      frame Default {
      }
      frame "Testing", "Safe" {
        w653 = T11."Enabled" ("Disabled")
        n163 = property on="Edit Fire \nSequence" class="Bool (strict)"() -> ("Value"=w655:bool)  [unwired: 2 in, 2 out]
        n164 = Select(t=w653, s=w655, f=T11."Disabled and Grayed Out" ("Disabled")) -> (s? t:f=w652:T11)
        n165 = Select(t=w653, s=w655, f=T11."Disabled" ("Disabled")) -> (s? t:f=w656:T11)
        n166 = property on="NC-F\nTiming" class="Slide (strict)"("DisabledEnum"=w656) -> ()  [unwired: 2 in, 2 out]
        n167 = property on="NC-FI\nTiming" class="Slide (strict)"("DisabledEnum"=w656) -> ()  [unwired: 2 in, 2 out]
        n168 = property on="NC-O\nTiming" class="Slide (strict)"("DisabledEnum"=w656) -> ()  [unwired: 2 in, 2 out]
        n169 = property on="NC-OI\nTiming" class="Slide (strict)"("DisabledEnum"=w656) -> ()  [unwired: 2 in, 2 out]
        n170 = property on="Ignitor\nTiming" class="Slide (strict)"("DisabledEnum"=w656) -> ()  [unwired: 2 in, 2 out]
        n171 = property on="Fire\nTiming" class="Slide (strict)"("DisabledEnum"=w656) -> ()  [unwired: 2 in, 2 out]
        n172 = property on="NC-F Invert" class="Bool (strict)"("DisabledEnum"=w652) -> ()  [unwired: 2 in, 2 out]
        n173 = property on="NC-FI Invert" class="Bool (strict)"("DisabledEnum"=w652) -> ()  [unwired: 2 in, 2 out]
        n174 = property on="NC-O Invert" class="Bool (strict)"("DisabledEnum"=w652) -> ()  [unwired: 2 in, 2 out]
        n175 = property on="NC-OI Invert" class="Bool (strict)"("DisabledEnum"=w652) -> ()  [unwired: 2 in, 2 out]
        n176 = property on="Ignitor Invert" class="Bool (strict)"("DisabledEnum"=w652) -> ()  [unwired: 2 in, 2 out]
        n177 = property on="Countdown + Fring\nLength" class="DigNum (strict)"("DisabledEnum"=w652) -> ()  [unwired: 2 in, 2 out]
        n178 = property on="NC-F Open Delay" class="DigNum (strict)"("DisabledEnum"=w652) -> ()  [unwired: 2 in, 2 out]
        n179 = property on="NC-FI Open Delay" class="DigNum (strict)"("DisabledEnum"=w652) -> ()  [unwired: 2 in, 2 out]
        n180 = property on="NC-O Open Delay" class="DigNum (strict)"("DisabledEnum"=w652) -> ()  [unwired: 2 in, 2 out]
        n181 = property on="NC-OI Open Delay" class="DigNum (strict)"("DisabledEnum"=w652) -> ()  [unwired: 2 in, 2 out]
        n182 = property on="Igniter Active Delay" class="DigNum (strict)"("DisabledEnum"=w652) -> ()  [unwired: 2 in, 2 out]
        n183 = property on="NC-F Close Delay" class="DigNum (strict)"("DisabledEnum"=w652) -> ()  [unwired: 2 in, 2 out]
        n184 = property on="NC-FI Close Delay" class="DigNum (strict)"("DisabledEnum"=w652) -> ()  [unwired: 2 in, 2 out]
        n185 = property on="NC-O Close Delay" class="DigNum (strict)"("DisabledEnum"=w652) -> ()  [unwired: 2 in, 2 out]
        n186 = property on="NC-OI Close Delay" class="DigNum (strict)"("DisabledEnum"=w652) -> ()  [unwired: 2 in, 2 out]
        n187 = property on="Igniter Inactive Delay" class="DigNum (strict)"("DisabledEnum"=w652) -> ()  [unwired: 2 in, 2 out]
      }
    }
    n188 = case shown="Default" w126 {
      tunnel: [w658 w659] -> w185
      tunnel: w171 -> [w658 _]
      frame "Firing" {
      }
      frame Default {
        n189 = Build Array("NC-F Invert", "NC-FI Invert", "NC-O Invert", "NC-OI Invert", "Ignitor Invert") -> (w666:bool[])
        n190 = Boolean To (0,1)(Boolean=w666) -> (0, 1=w667:i16[])
        n191 = Multiply(x=w667, y=2) -> (x*y=w659:i32[])
      }
    }
    n192 = feedback #3(i32[] [4, 4, 4, 4, 4]) -> (w198:i32[])
    n193 = feedback-in #3(w185) -> ()
    n194 = Not Equal?(x=w198, y=w185) -> (x != y?=w187:bool[])
    n195 = Index Array(array=w187, index #1=0 ("index"), index #2=1 ("index"), index #3=2 ("index"), index #4=3 ("index"), index #5=4 ("index")) -> (element #1=w186:bool, element #2=w182:bool, element #3=w181:bool, element #4=w180:bool, element #5=w179:bool)
    n196 = Index Array(array=w185, index #1=0 ("index"), index #2=1 ("index"), index #3=2 ("index"), index #4=3 ("index"), index #5=4 ("index")) -> (element #1=w183:i32, element #2=w184:i32, element #3=w178:i32, element #4=w177:i32, element #5=w176:i32)
    n197 = case shown="True" w186 {
      tunnel: w201 -> [_ w698]
      tunnel: w200 -> [_ w697]
      tunnel: w183 -> [_ w696]
      frame False {
      }
      frame True {
        n198 = for {
          N: w697 -> [_]
          tunnel: w698 -> [w702]
          tunnel: w696 -> [w699]
          i -> [w701]
          n199 = Index Array(array=w702, index (row)=w701, index (col)=w699) -> (element=w700:u32)
          n200 = property on="NC-F\nTiming" class="Slide (strict)"("Active Slider"=w701, "Fill Color"=w700) -> ()  [unwired: 2 in, 2 out]
        }
      }
    }
    n201 = case shown="True" w182 {
      tunnel: w201 -> [_ w691]
      tunnel: w200 -> [_ w690]
      tunnel: w184 -> [_ w689]
      frame False {
      }
      frame True {
        n202 = for {
          N: w690 -> [_]
          tunnel: w691 -> [w695]
          tunnel: w689 -> [w692]
          i -> [w694]
          n203 = Index Array(array=w695, index (row)=w694, index (col)=w692) -> (element=w693:u32)
          n204 = property on="NC-FI\nTiming" class="Slide (strict)"("Active Slider"=w694, "Fill Color"=w693) -> ()  [unwired: 2 in, 2 out]
        }
      }
    }
    n205 = case shown="True" w181 {
      tunnel: w201 -> [_ w684]
      tunnel: w200 -> [_ w683]
      tunnel: w178 -> [_ w682]
      frame False {
      }
      frame True {
        n206 = for {
          N: w683 -> [_]
          tunnel: w684 -> [w688]
          tunnel: w682 -> [w685]
          i -> [w687]
          n207 = Index Array(array=w688, index (row)=w687, index (col)=w685) -> (element=w686:u32)
          n208 = property on="NC-O\nTiming" class="Slide (strict)"("Active Slider"=w687, "Fill Color"=w686) -> ()  [unwired: 2 in, 2 out]
        }
      }
    }
    n209 = case shown="True" w180 {
      tunnel: w201 -> [_ w677]
      tunnel: w200 -> [_ w676]
      tunnel: w177 -> [_ w675]
      frame False {
      }
      frame True {
        n210 = for {
          N: w676 -> [_]
          tunnel: w677 -> [w681]
          tunnel: w675 -> [w678]
          i -> [w680]
          n211 = Index Array(array=w681, index (row)=w680, index (col)=w678) -> (element=w679:u32)
          n212 = property on="NC-OI\nTiming" class="Slide (strict)"("Active Slider"=w680, "Fill Color"=w679) -> ()  [unwired: 2 in, 2 out]
        }
      }
    }
    n213 = case shown="True" w179 {
      tunnel: w201 -> [_ w670]
      tunnel: w200 -> [_ w669]
      tunnel: w176 -> [_ w668]
      frame False {
      }
      frame True {
        n214 = for {
          N: w669 -> [_]
          tunnel: w670 -> [w674]
          tunnel: w668 -> [w671]
          i -> [w673]
          n215 = Index Array(array=w674, index (row)=w673, index (col)=w671) -> (element=w672:u32)
          n216 = property on="Ignitor\nTiming" class="Slide (strict)"("Active Slider"=w673, "Fill Color"=w672) -> ()  [unwired: 2 in, 2 out]
        }
      }
    }
    n217 = call <vilib>:"High Resolution Relative Seconds.vi"() -> ("relative seconds"=w224:dbl)
    n218 = feedback-in #4(w224) -> ()
    n219 = feedback #4(w224) -> (w215:dbl)
    n220 = case shown="False" "Pause DAQ" {
      tunnel: [w271 T10."Pause" ("SetState")] -> w147
      frame False {
        # "DAQ is unpaused:\nallow recording and overdrive"
        n221 = case shown="True" "Record" {
          tunnel: [T10."Default" ("SetState") w274] -> w271
          frame False {
            n222 = property on="Overdrive" class="Bool (strict)"("Value"=FALSE) -> ()  [unwired: 2 in, 2 out]
          }
          frame True {
            n223 = Select(t=T10."Overdrive" ("SetState"), s="Overdrive", f=T10."Record" ("SetState")) -> (s? t:f=w274:T10)
          }
        }
      }
      frame True {
        # "Pause DAQ"
      }
    }
    n224 = Subtract(x=w224, y=w215) -> (x-y=w222:dbl)
    n225 = feedback #5(0.0) -> (w221:dbl)
    n226 = case shown="True" "Pump" {
      tunnel: w222 -> [_ w925]
      tunnel: w221 -> [w923 w926]
      tunnel: [w923 w924] -> w217
      frame False {
      }
      frame True {
        n227 = Add(x=w925, y=w926) -> (x+y=w924:dbl)
      }
    }
    n228 = Equal To 0?(x="Ignition Type") -> (x = 0?=w157:bool)
    n229 = Equal?(x=T1."Firing" ("System State"), y=w126) -> (x = y?=w158:bool)
    n230 = Equal To 0?(x="Ignition Type (Testing)") -> (x = 0?=w165:bool)
    n231 = And(x="Ignition ARM (Testing)", y=w165) -> (x .and. y?=w160:bool)
    n232 = And(x=w157, y=w158) -> (x .and. y?=w159:bool)
    n233 = Select(t=0.0 ("f"), s="Reset Timer", f=w217) -> (s? t:f=w219:dbl)
    "Fill Progress" <- w219
    "Fill Timer" <- w219
    n234 = feedback-in #5(w219) -> ()
    n235 = property on="Fill Progress" class="Slide (strict)"("Scale.Maximum"="Time Target", "Scale.Minimum"=0.0 ("Scale.Range:Minimum")) -> ()  [unwired: 2 in, 2 out]
    n236 = Or(x=w160, y=w159) -> (x .or. y?=w135:bool)
    n237 = Less Or Equal?(x="Time Target", y=w219) -> (x <= y?=w170:bool)
    n238 = call "Is Value Changed.vim"("value"=w147) -> ("changed or first call?"=w148:bool)
    n239 = case shown="True" "Ignition ARM (Testing)" {
      tunnel: "Ignition Type (Testing)" -> [_ w917]
      frame False {
        w913 = T11."Enabled" ("Disabled")
        # "Ignition Test SAFE:\n-Disable igniton test and set to 0\n-Enable changing ignition type\n-Enable NC-FP and NC-OP Actuation"
        n240 = property on="Ignition Type (Testing)" class="Ring (strict)"("DisabledEnum"=T11."Enabled" ("Disabled")) -> ()  [unwired: 2 in, 2 out]
        n241 = property on="Ignition\nTest" class="Bool (strict)"("DisabledEnum"=T11."Disabled and Grayed Out" ("Disabled"), "Value"=FALSE ("Pump")) -> ()  [unwired: 2 in, 2 out]
        n242 = property on="NC-FP" class="Bool (strict)"("DisabledEnum"=w913) -> ()  [unwired: 2 in, 2 out]
        n243 = property on="NC-OP" class="Bool (strict)"("DisabledEnum"=w913) -> ()  [unwired: 2 in, 2 out]
      }
      frame True {
        # "Ignition Test ARMED:\n-Enable ignition test controls\n-Disable changing ignition type\n-Disable NC-FP and NC-OP actuation if Spark Plug is selected"
        n244 = case shown="0" w917 {
          frame 0 {
            w920 = FALSE
            w921 = T11."Disabled and Grayed Out" ("Disabled")
            n245 = property on="NC-FP" class="Bool (strict)"("DisabledEnum"=w921, "Value"=w920) -> ()  [unwired: 2 in, 2 out]
            n246 = property on="NC-OP" class="Bool (strict)"("DisabledEnum"=w921, "Value"=w920) -> ()  [unwired: 2 in, 2 out]
          }
          frame 1, 2, Default {
            w922 = T11."Enabled" ("Disabled")
            n247 = property on="NC-OP" class="Bool (strict)"("DisabledEnum"=w922) -> ()  [unwired: 2 in, 2 out]
            n248 = property on="NC-FP" class="Bool (strict)"("DisabledEnum"=w922) -> ()  [unwired: 2 in, 2 out]
          }
        }
        n249 = property on="Ignition\nTest" class="Bool (strict)"("DisabledEnum"=T11."Enabled" ("Disabled")) -> ()  [unwired: 2 in, 2 out]
        n250 = property on="Ignition Type (Testing)" class="Ring (strict)"("DisabledEnum"=T11."Disabled and Grayed Out" ("Disabled")) -> ()  [unwired: 2 in, 2 out]
      }
    }
    n251 = case shown="True" w148 {
      tunnel: w147 -> [_ w268]
      tunnel: w146 -> [_ w265]
      tunnel: w145 -> [_ w266]
      frame False {
        # "Maintain previous\nstates"
      }
      frame True {
        w269 = string[] ["Default", "Record", "Overdrive", "Pause"]  # DAQ Messages
        # "Pass new states along\nto DAQ whenever\nthey are updated"
        n252 = Index Array(array=w269, index=w268) -> (element=w267:string)
        n253 = Send Notification(notification=w267, notifier=w265) -> ()  [unwired: 1 in, 2 out]
        n254 = Send Notification(notification=w267, notifier=w266) -> ()  [unwired: 1 in, 2 out]
      }
    }
    n255 = case shown="True" w170 {
      frame False {
        # "Default case; timer has not reached its target and pressure is safe for pumping:\n-enable pump controls"
        n256 = property on="Pump" class="Bool (strict)"("DisabledEnum"=T11."Enabled" ("Disabled")) -> ()  [unwired: 2 in, 2 out]
      }
      frame True {
        # "Timer has reached its target -OR- PT-1F pressure is too high for safe pump operation:\ndisable pump controls"
        n257 = property on="Pump" class="Bool (strict)"("DisabledEnum"=T11."Disabled and Grayed Out" ("Disabled"), "Value"=FALSE ("Pump")) -> ()  [unwired: 2 in, 2 out]
      }
    }
    n258 = property on="Pump" class="Bool (strict)"() -> ("Value"=w140:bool)  [unwired: 2 in, 2 out]
    n259 = Or(x="Ignition\nTest", y=w162) -> (x .or. y?=w144:bool)
    n260 = property on="Record" class="Bool (strict)"() -> ("Value"=w133:bool)  [unwired: 2 in, 2 out]
    "RecordStatus" <- w133
    n261 = Boolean To (0,1)(Boolean=w140) -> (0, 1=w129:i16)
    n262 = Boolean To (0,1)(Boolean=w135) -> (0, 1=w128:i16)
    n263 = Boolean To (0,1)(Boolean=w144) -> (0, 1=w127:i16)
    n264 = call "DigitalOut_2.vi"("Purge Valves"=w163, "Spark Arm"=w135, "Ignition!"=w144) -> ("purge valves out"=w136:bool[])  [unwired: 8 in]
    n265 = Insert Into Array(array=w143, new element=w136) -> (w139:bool[])  [unwired: 1 in]
    n266 = Boolean Array To Number(Boolean array=w139) -> (number=w130:u32)
    n267 = Merge Signals(w130, w129, w128, w127, w126) -> (w141:dynamicdata)
    n268 = Build Array(w130, w129, w128, w127, w126) -> (w125:u32[])
    n269 = Get Date/Time In Seconds() -> (seconds since 1Jan1904=w134:timestamp)
    n270 = call "Is Value Changed.vim"("value"=w125) -> ("changed or first call?"=w138:bool)
    n271 = feedback #6() -> (w132:timestamp)  [unwired: 1 in]
    n272 = case shown="True" w133 {
      tunnel: w132 -> [w226 w229]
      tunnel: [w226 w228] -> w131
      frame False {
      }
      frame True {
        n273 = First Call?() -> (First Call?: T/F=w227:bool)
        n274 = case shown="True" w227 {
          tunnel: [w230 w231] -> w228
          tunnel: w229 -> [w230 _]
          frame False {
          }
          frame True {
            n275 = Get Date/Time In Seconds() -> (seconds since 1Jan1904=w231:timestamp)
          }
        }
      }
    }
    n276 = feedback-in #6(w131) -> ()
    n277 = And(x=w133, y=w138) -> (x .and. y?=w137:bool)
    n278 = Insert Into Array(array=w143, new element="Pump") -> (w168:bool[])  [unwired: 1 in]
    n279 = case shown="True" w153 {
      tunnel: w168 -> [_ w289]
      tunnel: w136 -> [_ w288]
      tunnel: w152 -> [_ w284]
      tunnel: w151 -> [_ w285]
      frame False {
      }
      frame True {
        # "This conditional box from left to right:\n-First IF conditional: control the positions of the sliders in the\ntiming sequence to match the desired hardware delays.\n- The sensor and load cell data is gathered and conditioned\nto reduce noise, and warning/error thresholds are gathered\nfrom the GUI\n- FOR loop: determine whether sensor data is within error\nranges and set UI colors accordingly\n- Pass sensor data, valve data, and error states along to the\nP&ID GUI vi for further display."
        # "Update most of the readouts at a relatively low rate - all of these display ops take a long time to process"
        n280 = case shown="True" "Edit Fire \nSequence" {
          frame False {
          }
          frame True {
            n281 = Unbundle("NC-F\nTiming") -> (w314:dbl, w313:dbl, w312:dbl, w311:dbl)  [unwired: 2 out]
            n282 = Unbundle("NC-FI\nTiming") -> (w321:dbl, w320:dbl, w319:dbl, w318:dbl)  [unwired: 2 out]
            n283 = Unbundle("NC-O\nTiming") -> (w327:dbl, w326:dbl, w325:dbl, w324:dbl)  [unwired: 2 out]
            n284 = Subtract(x=w313, y="NC-F Open Delay") -> (x-y=w310:dbl)
            n285 = Subtract(x=w312, y="NC-F Close Delay") -> (x-y=w309:dbl)
            n286 = Subtract(x=w320, y="NC-FI Open Delay") -> (x-y=w317:dbl)
            n287 = Subtract(x=w319, y="NC-FI Close Delay") -> (x-y=w316:dbl)
            n288 = Subtract(x=w326, y="NC-O Open Delay") -> (x-y=w323:dbl)
            n289 = Subtract(x=w325, y="NC-O Close Delay") -> (x-y=w322:dbl)
            n290 = Bundle(w314, w310, w313, w309, w312, w311) -> (w308:cluster{dbl, dbl, dbl, dbl, dbl, dbl})  [unwired: 1 in]
            n291 = Bundle(w321, w317, w320, w316, w319, w318) -> (w352:cluster{dbl, dbl, dbl, dbl, dbl, dbl})  [unwired: 1 in]
            n292 = Bundle(w327, w323, w326, w322, w325, w324) -> (w353:cluster{dbl, dbl, dbl, dbl, dbl, dbl})  [unwired: 1 in]
            n293 = property on="Countdown + Firing\nLength" class="DigNum (strict)"() -> ("Value"=w304:dbl)  [unwired: 2 in, 2 out]
            n294 = property on="NC-F\nTiming" class="Slide (strict)"("Value"=w308, "Scale.Maximum"=w304) -> ()  [unwired: 2 in, 2 out]
            n295 = property on="NC-FI\nTiming" class="Slide (strict)"("Value"=w352, "Scale.Maximum"=w304) -> ()  [unwired: 2 in, 2 out]
            n296 = property on="NC-O\nTiming" class="Slide (strict)"("Value"=w353, "Scale.Maximum"=w304) -> ()  [unwired: 2 in, 2 out]
            n297 = Unbundle("NC-OI\nTiming") -> (w333:dbl, w332:dbl, w331:dbl, w330:dbl)  [unwired: 2 out]
            n298 = Unbundle("Ignitor\nTiming") -> (w339:dbl, w338:dbl, w337:dbl, w336:dbl)  [unwired: 2 out]
            n299 = Subtract(x=w332, y="NC-OI Open Delay") -> (x-y=w329:dbl)
            n300 = Subtract(x=w331, y="NC-OI Close Delay") -> (x-y=w328:dbl)
            n301 = Subtract(x=w338, y="Igniter Active Delay") -> (x-y=w335:dbl)
            n302 = Subtract(x=w337, y="Igniter Inactive Delay") -> (x-y=w334:dbl)
            n303 = Bundle(w333, w329, w332, w328, w331, w330) -> (w354:cluster{dbl, dbl, dbl, dbl, dbl, dbl})  [unwired: 1 in]
            n304 = Bundle(w339, w335, w338, w334, w337, w336) -> (w355:cluster{dbl, dbl, dbl, dbl, dbl, dbl})  [unwired: 1 in]
            n305 = property on="NC-OI\nTiming" class="Slide (strict)"("Value"=w354, "Scale.Maximum"=w304) -> ()  [unwired: 2 in, 2 out]
            n306 = property on="Ignitor\nTiming" class="Slide (strict)"("Value"=w355, "Scale.Maximum"=w304) -> ()  [unwired: 2 in, 2 out]
            n307 = property on="Fire\nTiming" class="Slide (strict)"("Value"="Fire\nTiming", "Scale.Maximum"=w304) -> ()  [unwired: 2 in, 2 out]
          }
        }
        n308 = call "ProcessSignals.vi"("UI Queue"=w284) -> ("Array"=w281:dbl[])  [unwired: 9 in, 1 out]
        n309 = call "ProcessSignals.vi"("UI Queue"=w285) -> ("Array"=w286:dbl[])  [unwired: 9 in, 1 out]
        n310 = Insert Into Array(array=w281, new element=w286) -> (w282:dbl[])  [unwired: 1 in]
        n311 = Insert Into Array(array="Warning 1", new element #1="Warning 2", new element #2="Warning 3", new element #3="Warning 4") -> (w300:dbl[])  [unwired: 1 in]
        n312 = Insert Into Array(array="Error 1", new element #1="Error 2", new element #2="Error 3", new element #3="Error 4") -> (w299:dbl[])  [unwired: 1 in]
        n313 = Array Size(array=w282) -> (size(s)=w283:i32)
        n314 = for {
          N: w283 -> [_]
          tunnel: w300 -> [w357] mode=indexing
          tunnel: w299 -> [w363] mode=indexing
          tunnel: w282 -> [w358] mode=indexing
          tunnel: [w362] -> w279 mode=indexing
          tunnel: [w361] -> w292 mode=indexing
          tunnel: [w360] -> w293 mode=indexing
          tunnel: [w359] -> w291 mode=indexing
          i -> [w367]
          w364 = u32[] [0, 0, 0, 16776960]  # Text Colors
          w365 = u32[] [13816530, 65280, 16776960, 16711680]  # BG Colors
          n315 = Greater?(x=w358, y=w363) -> (0:w366:bool)
          n316 = Less?(x=w357, y=w358) -> (x < y?=w356:bool)
          n317 = case shown="21" w367 {
            tunnel: w356 -> [w370 w379 w392 w405 w418 w431 w444 w457 w470 w483 w496 w509 w522 w535 w549 w561 w573 w585 w597 w609 w620 w633 w646]
            tunnel: w366 -> [w371 w378 w391 w404 w417 w430 w443 w456 w469 w482 w495 w508 w521 w534 w548 w560 w572 w584 w596 w608 w619 w632 w645]
            tunnel: w365 -> [_ w377 w390 w403 w416 w429 w442 w455 w468 w481 w494 w507 w520 w533 w547 w559 w571 w583 w595 w607 w618 w631 w644]
            tunnel: w364 -> [_ w374 w387 w400 w413 w426 w439 w452 w465 w478 w491 w504 w517 w530 w544 w556 w568 w580 w592 w604 w615 w628 w641]
            tunnel: [w371 w378 w391 w404 w417 w430 w443 w456 w469 w482 w495 w508 w521 w534 w548 w560 w572 w584 w596 w608 w619 w632 w645] -> w362
            tunnel: [w370 w379 w392 w405 w418 w431 w444 w457 w470 w483 w496 w509 w522 w535 w549 w561 w573 w585 w597 w609 w620 w633 w646] -> w361
            tunnel: w358 -> [w369 w372 w385 w398 w411 w424 w437 w450 w463 w476 w489 w502 w515 w528 w542 w554 w566 w578 w590 w602 w613 w626 w639]
            tunnel: [w369 w372 w385 w398 w411 w424 w437 w450 w463 w476 w489 w502 w515 w528 w542 w554 w566 w578 w590 w602 w613 w626 w639] -> w360
            tunnel: [FALSE w380 w393 w406 w419 w432 w445 w458 w471 w484 w497 w510 w523 w536 w541 w553 w565 w577 w589 w601 w621 w634 w647] -> w359
            frame Default {
            }
            frame 0 {
              n318 = Greater?(x=w372, y=10.0) -> (0:w380:bool)
              n319 = Boolean To (0,1)(Boolean=w380) -> (0, 1=w383:i16)
              n320 = Boolean To (0,1)(Boolean=w378) -> (0, 1=w381:i16)
              n321 = Boolean To (0,1)(Boolean=w379) -> (0, 1=w382:i16)
              n322 = Compound Arithmetic op=ADD(w383, w381, w382) -> (w373:i16)
              n323 = Index Array(array=w377, index=w373) -> (element=w376:u32)
              n324 = Index Array(array=w374, index=w373) -> (element=w375:u32)
              n325 = property on="PT-1P" class="DigNum (strict)"("NumText.BGColor"=w376, "NumText.TextColor"=w375) -> ()  [unwired: 2 in, 2 out]
              "PT-1P" <- w372
            }
            frame 1 {
              n326 = Greater?(x=w385, y=10.0) -> (0:w393:bool)
              n327 = Boolean To (0,1)(Boolean=w393) -> (0, 1=w396:i16)
              n328 = Boolean To (0,1)(Boolean=w391) -> (0, 1=w394:i16)
              n329 = Boolean To (0,1)(Boolean=w392) -> (0, 1=w395:i16)
              n330 = Compound Arithmetic op=ADD(w396, w394, w395) -> (w386:i16)
              n331 = Index Array(array=w390, index=w386) -> (element=w389:u32)
              n332 = Index Array(array=w387, index=w386) -> (element=w388:u32)
              n333 = property on="PT-2P" class="DigNum (strict)"("NumText.BGColor"=w389, "NumText.TextColor"=w388) -> ()  [unwired: 2 in, 2 out]
              "PT-2P" <- w385
            }
            frame 2 {
              n334 = Greater?(x=w398, y=10.0) -> (0:w406:bool)
              n335 = Boolean To (0,1)(Boolean=w406) -> (0, 1=w409:i16)
              n336 = Boolean To (0,1)(Boolean=w404) -> (0, 1=w407:i16)
              n337 = Boolean To (0,1)(Boolean=w405) -> (0, 1=w408:i16)
              n338 = Compound Arithmetic op=ADD(w409, w407, w408) -> (w399:i16)
              n339 = Index Array(array=w403, index=w399) -> (element=w402:u32)
              n340 = Index Array(array=w400, index=w399) -> (element=w401:u32)
              n341 = property on="PT-3P" class="DigNum (strict)"("NumText.BGColor"=w402, "NumText.TextColor"=w401) -> ()  [unwired: 2 in, 2 out]
              "PT-3P" <- w398
            }
            frame 3 {
              n342 = Greater?(x=w411, y=10.0) -> (0:w419:bool)
              n343 = Boolean To (0,1)(Boolean=w419) -> (0, 1=w422:i16)
              n344 = Boolean To (0,1)(Boolean=w417) -> (0, 1=w420:i16)
              n345 = Boolean To (0,1)(Boolean=w418) -> (0, 1=w421:i16)
              n346 = Compound Arithmetic op=ADD(w422, w420, w421) -> (w412:i16)
              n347 = Index Array(array=w416, index=w412) -> (element=w415:u32)
              n348 = Index Array(array=w413, index=w412) -> (element=w414:u32)
              n349 = property on="PT-1F" class="DigNum (strict)"("NumText.BGColor"=w415, "NumText.TextColor"=w414) -> ()  [unwired: 2 in, 2 out]
              "PT-1F" <- w411
            }
            frame 4 {
              n350 = Greater?(x=w424, y=10.0) -> (0:w432:bool)
              n351 = Boolean To (0,1)(Boolean=w432) -> (0, 1=w435:i16)
              n352 = Boolean To (0,1)(Boolean=w430) -> (0, 1=w433:i16)
              n353 = Boolean To (0,1)(Boolean=w431) -> (0, 1=w434:i16)
              n354 = Compound Arithmetic op=ADD(w435, w433, w434) -> (w425:i16)
              n355 = Index Array(array=w429, index=w425) -> (element=w428:u32)
              n356 = Index Array(array=w426, index=w425) -> (element=w427:u32)
              n357 = property on="PT-1O" class="DigNum (strict)"("NumText.BGColor"=w428, "NumText.TextColor"=w427) -> ()  [unwired: 2 in, 2 out]
              "PT-1O" <- w424
            }
            frame 5 {
              n358 = Greater?(x=w437, y=10.0) -> (0:w445:bool)
              n359 = Boolean To (0,1)(Boolean=w445) -> (0, 1=w448:i16)
              n360 = Boolean To (0,1)(Boolean=w443) -> (0, 1=w446:i16)
              n361 = Boolean To (0,1)(Boolean=w444) -> (0, 1=w447:i16)
              n362 = Compound Arithmetic op=ADD(w448, w446, w447) -> (w438:i16)
              n363 = Index Array(array=w442, index=w438) -> (element=w441:u32)
              n364 = Index Array(array=w439, index=w438) -> (element=w440:u32)
              n365 = property on="PT-2O" class="DigNum (strict)"("NumText.BGColor"=w441, "NumText.TextColor"=w440) -> ()  [unwired: 2 in, 2 out]
              "PT-2O" <- w437
            }
            frame 6 {
              n366 = Greater?(x=w450, y=10.0) -> (0:w458:bool)
              n367 = Boolean To (0,1)(Boolean=w458) -> (0, 1=w461:i16)
              n368 = Boolean To (0,1)(Boolean=w456) -> (0, 1=w459:i16)
              n369 = Boolean To (0,1)(Boolean=w457) -> (0, 1=w460:i16)
              n370 = Compound Arithmetic op=ADD(w461, w459, w460) -> (w451:i16)
              n371 = Index Array(array=w455, index=w451) -> (element=w454:u32)
              n372 = Index Array(array=w452, index=w451) -> (element=w453:u32)
              n373 = property on="PT-FI" class="DigNum (strict)"("NumText.BGColor"=w454, "NumText.TextColor"=w453) -> ()  [unwired: 2 in, 2 out]
              "PT-FI" <- w450
            }
            frame 7 {
              n374 = Greater?(x=w463, y=10.0) -> (0:w471:bool)
              n375 = Boolean To (0,1)(Boolean=w471) -> (0, 1=w474:i16)
              n376 = Boolean To (0,1)(Boolean=w469) -> (0, 1=w472:i16)
              n377 = Boolean To (0,1)(Boolean=w470) -> (0, 1=w473:i16)
              n378 = Compound Arithmetic op=ADD(w474, w472, w473) -> (w464:i16)
              n379 = Index Array(array=w468, index=w464) -> (element=w467:u32)
              n380 = Index Array(array=w465, index=w464) -> (element=w466:u32)
              n381 = property on="PT-OI" class="DigNum (strict)"("NumText.BGColor"=w467, "NumText.TextColor"=w466) -> ()  [unwired: 2 in, 2 out]
              "PT-OI" <- w463
            }
            frame 8 {
              n382 = Greater?(x=w476, y=10.0) -> (0:w484:bool)
              n383 = Boolean To (0,1)(Boolean=w484) -> (0, 1=w487:i16)
              n384 = Boolean To (0,1)(Boolean=w482) -> (0, 1=w485:i16)
              n385 = Boolean To (0,1)(Boolean=w483) -> (0, 1=w486:i16)
              n386 = Compound Arithmetic op=ADD(w487, w485, w486) -> (w477:i16)
              n387 = Index Array(array=w481, index=w477) -> (element=w480:u32)
              n388 = Index Array(array=w478, index=w477) -> (element=w479:u32)
              n389 = property on="PT-CI" class="DigNum (strict)"("NumText.BGColor"=w480, "NumText.TextColor"=w479) -> ()  [unwired: 2 in, 2 out]
              "PT-CI" <- w476
            }
            frame 9 {
              n390 = Greater?(x=w489, y=10.0) -> (0:w497:bool)
              n391 = Boolean To (0,1)(Boolean=w497) -> (0, 1=w500:i16)
              n392 = Boolean To (0,1)(Boolean=w495) -> (0, 1=w498:i16)
              n393 = Boolean To (0,1)(Boolean=w496) -> (0, 1=w499:i16)
              n394 = Compound Arithmetic op=ADD(w500, w498, w499) -> (w490:i16)
              n395 = Index Array(array=w494, index=w490) -> (element=w493:u32)
              n396 = Index Array(array=w491, index=w490) -> (element=w492:u32)
              n397 = property on="PT-1E" class="DigNum (strict)"("NumText.BGColor"=w493, "NumText.TextColor"=w492) -> ()  [unwired: 2 in, 2 out]
              "PT-1E" <- w489
            }
            frame 10 {
              n398 = Greater?(x=w502, y=10.0) -> (0:w510:bool)
              n399 = Boolean To (0,1)(Boolean=w510) -> (0, 1=w513:i16)
              n400 = Boolean To (0,1)(Boolean=w508) -> (0, 1=w511:i16)
              n401 = Boolean To (0,1)(Boolean=w509) -> (0, 1=w512:i16)
              n402 = Compound Arithmetic op=ADD(w513, w511, w512) -> (w503:i16)
              n403 = Index Array(array=w507, index=w503) -> (element=w506:u32)
              n404 = Index Array(array=w504, index=w503) -> (element=w505:u32)
              n405 = property on="PT-2E" class="DigNum (strict)"("NumText.BGColor"=w506, "NumText.TextColor"=w505) -> ()  [unwired: 2 in, 2 out]
              "PT-2E" <- w502
            }
            frame 11 {
              n406 = Greater?(x=w515, y=10.0) -> (0:w523:bool)
              n407 = Boolean To (0,1)(Boolean=w523) -> (0, 1=w526:i16)
              n408 = Boolean To (0,1)(Boolean=w521) -> (0, 1=w524:i16)
              n409 = Boolean To (0,1)(Boolean=w522) -> (0, 1=w525:i16)
              n410 = Compound Arithmetic op=ADD(w526, w524, w525) -> (w516:i16)
              n411 = Index Array(array=w520, index=w516) -> (element=w519:u32)
              n412 = Index Array(array=w517, index=w516) -> (element=w518:u32)
              n413 = property on="PT-3E" class="DigNum (strict)"("NumText.BGColor"=w519, "NumText.TextColor"=w518) -> ()  [unwired: 2 in, 2 out]
              "PT-3E" <- w515
            }
            frame 12 {
              n414 = Greater?(x=w528, y=10.0) -> (0:w536:bool)
              n415 = Boolean To (0,1)(Boolean=w536) -> (0, 1=w539:i16)
              n416 = Boolean To (0,1)(Boolean=w534) -> (0, 1=w537:i16)
              n417 = Boolean To (0,1)(Boolean=w535) -> (0, 1=w538:i16)
              n418 = Compound Arithmetic op=ADD(w539, w537, w538) -> (w529:i16)
              n419 = Index Array(array=w533, index=w529) -> (element=w532:u32)
              n420 = Index Array(array=w530, index=w529) -> (element=w531:u32)
              n421 = property on="PT-L" class="DigNum (strict)"("NumText.BGColor"=w532, "NumText.TextColor"=w531) -> ()  [unwired: 2 in, 2 out]
              "PT-L" <- w528
            }
            frame 13 {
              w541 = TRUE
              n422 = Boolean To (0,1)(Boolean=w541) -> (0, 1=w552:i16)
              n423 = Boolean To (0,1)(Boolean=w548) -> (0, 1=w550:i16)
              n424 = Boolean To (0,1)(Boolean=w549) -> (0, 1=w551:i16)
              n425 = Compound Arithmetic op=ADD(w552, w550, w551) -> (w543:i16)
              n426 = Index Array(array=w547, index=w543) -> (element=w546:u32)
              n427 = Index Array(array=w544, index=w543) -> (element=w545:u32)
              n428 = property on="TC-1P" class="DigNum (strict)"("NumText.BGColor"=w546, "NumText.TextColor"=w545) -> ()  [unwired: 2 in, 2 out]
              "TC-1P" <- w542
            }
            frame 14 {
              w553 = TRUE
              n429 = Boolean To (0,1)(Boolean=w553) -> (0, 1=w564:i16)
              n430 = Boolean To (0,1)(Boolean=w560) -> (0, 1=w562:i16)
              n431 = Boolean To (0,1)(Boolean=w561) -> (0, 1=w563:i16)
              n432 = Compound Arithmetic op=ADD(w564, w562, w563) -> (w555:i16)
              n433 = Index Array(array=w559, index=w555) -> (element=w558:u32)
              n434 = Index Array(array=w556, index=w555) -> (element=w557:u32)
              n435 = property on="TC-2P" class="DigNum (strict)"("NumText.BGColor"=w558, "NumText.TextColor"=w557) -> ()  [unwired: 2 in, 2 out]
              "TC-2P" <- w554
            }
            frame 15 {
              w565 = TRUE
              n436 = Boolean To (0,1)(Boolean=w565) -> (0, 1=w576:i16)
              n437 = Boolean To (0,1)(Boolean=w572) -> (0, 1=w574:i16)
              n438 = Boolean To (0,1)(Boolean=w573) -> (0, 1=w575:i16)
              n439 = Compound Arithmetic op=ADD(w576, w574, w575) -> (w567:i16)
              n440 = Index Array(array=w571, index=w567) -> (element=w570:u32)
              n441 = Index Array(array=w568, index=w567) -> (element=w569:u32)
              n442 = property on="TC-3P" class="DigNum (strict)"("NumText.BGColor"=w570, "NumText.TextColor"=w569) -> ()  [unwired: 2 in, 2 out]
              "TC-3P" <- w566
            }
            frame 16 {
              w577 = TRUE
              n443 = Boolean To (0,1)(Boolean=w577) -> (0, 1=w588:i16)
              n444 = Boolean To (0,1)(Boolean=w584) -> (0, 1=w586:i16)
              n445 = Boolean To (0,1)(Boolean=w585) -> (0, 1=w587:i16)
              n446 = Compound Arithmetic op=ADD(w588, w586, w587) -> (w579:i16)
              n447 = Index Array(array=w583, index=w579) -> (element=w582:u32)
              n448 = Index Array(array=w580, index=w579) -> (element=w581:u32)
              n449 = property on="TC-1F" class="DigNum (strict)"("NumText.BGColor"=w582, "NumText.TextColor"=w581) -> ()  [unwired: 2 in, 2 out]
              "TC-1F" <- w578
            }
            frame 17 {
              w589 = TRUE
              n450 = Boolean To (0,1)(Boolean=w589) -> (0, 1=w600:i16)
              n451 = Boolean To (0,1)(Boolean=w596) -> (0, 1=w598:i16)
              n452 = Boolean To (0,1)(Boolean=w597) -> (0, 1=w599:i16)
              n453 = Compound Arithmetic op=ADD(w600, w598, w599) -> (w591:i16)
              n454 = Index Array(array=w595, index=w591) -> (element=w594:u32)
              n455 = Index Array(array=w592, index=w591) -> (element=w593:u32)
              n456 = property on="TC-1O" class="DigNum (strict)"("NumText.BGColor"=w594, "NumText.TextColor"=w593) -> ()  [unwired: 2 in, 2 out]
              "TC-1O" <- w590
            }
            frame 18 {
              w601 = TRUE
              n457 = Boolean To (0,1)(Boolean=w601) -> (0, 1=w612:i16)
              n458 = Boolean To (0,1)(Boolean=w608) -> (0, 1=w610:i16)
              n459 = Boolean To (0,1)(Boolean=w609) -> (0, 1=w611:i16)
              n460 = Compound Arithmetic op=ADD(w612, w610, w611) -> (w603:i16)
              n461 = Index Array(array=w607, index=w603) -> (element=w606:u32)
              n462 = Index Array(array=w604, index=w603) -> (element=w605:u32)
              n463 = property on="TC-2O" class="DigNum (strict)"("NumText.BGColor"=w606, "NumText.TextColor"=w605) -> ()  [unwired: 2 in, 2 out]
              "TC-2O" <- w602
            }
            frame 19 {
              n464 = Greater?(x=w613, y=0.5) -> (0:w621:bool)
              n465 = Boolean To (0,1)(Boolean=w621) -> (0, 1=w624:i16)
              n466 = Boolean To (0,1)(Boolean=w619) -> (0, 1=w622:i16)
              n467 = Boolean To (0,1)(Boolean=w620) -> (0, 1=w623:i16)
              n468 = Compound Arithmetic op=ADD(w624, w622, w623) -> (w614:i16)
              n469 = Index Array(array=w618, index=w614) -> (element=w617:u32)
              n470 = Index Array(array=w615, index=w614) -> (element=w616:u32)
              n471 = property on="FM-F" class="DigNum (strict)"("NumText.BGColor"=w617, "NumText.TextColor"=w616) -> ()  [unwired: 2 in, 2 out]
              "FM-F" <- w613
            }
            frame 20 {
              n472 = Greater?(x=w626, y=10.0) -> (0:w634:bool)
              n473 = Boolean To (0,1)(Boolean=w634) -> (0, 1=w637:i16)
              n474 = Boolean To (0,1)(Boolean=w632) -> (0, 1=w635:i16)
              n475 = Boolean To (0,1)(Boolean=w633) -> (0, 1=w636:i16)
              n476 = Compound Arithmetic op=ADD(w637, w635, w636) -> (w627:i16)
              n477 = Index Array(array=w631, index=w627) -> (element=w630:u32)
              n478 = Index Array(array=w628, index=w627) -> (element=w629:u32)
              n479 = property on="FM-O" class="DigNum (strict)"("NumText.BGColor"=w630, "NumText.TextColor"=w629) -> ()  [unwired: 2 in, 2 out]
              "FM-O" <- w626
            }
            frame 21 {
              n480 = Greater?(x=w639, y=10.0) -> (0:w647:bool)
              n481 = Boolean To (0,1)(Boolean=w647) -> (0, 1=w650:i16)
              n482 = Boolean To (0,1)(Boolean=w645) -> (0, 1=w648:i16)
              n483 = Boolean To (0,1)(Boolean=w646) -> (0, 1=w649:i16)
              n484 = Compound Arithmetic op=ADD(w650, w648, w649) -> (w640:i16)
              n485 = Index Array(array=w644, index=w640) -> (element=w643:u32)
              n486 = Index Array(array=w641, index=w640) -> (element=w642:u32)
              n487 = property on="LC-E" class="DigNum (strict)"("NumText.BGColor"=w643, "NumText.TextColor"=w642) -> ()  [unwired: 2 in, 2 out]
              "LC-E" <- w639
            }
          }
        }
        n488 = Or Array Elements(Boolean array=w279) -> (logical OR=→"ERROR":bool)
        n489 = Insert Into Array(array=w289, new element=w288) -> (w290:bool[])  [unwired: 1 in]
        n490 = call "P&ID.vi"("Valves"=w290, "Errors"=w279, "Warnings"=w292, "HasReadings"=w291, "Readings"=w293) -> ()  [unwired: 7 in]
      }
    }
    n491 = case shown="True" w137 {
      tunnel: w141 -> [_ w238]
      tunnel: w134 -> [_ w237]
      tunnel: w142 -> [_ w235]
      tunnel: w131 -> [_ w232]
      frame False {
        # "No need to save data when nothing has changed\n(or when we're not recording)"
      }
      frame True {
        w234 = string[] ["Valves", "Pump", "Spark Arm", "Ignition", "Sytem State"]
        # "Add to output queue"
        # "Whever the valves, ignition, pump, or system\nstate changes while recording, save it to file"
        n492 = Array Size(array=w234) -> (size(s)=w233:i32)
        n493 = for {
          N: w233 -> [_]
          shift-right: [w243] -> w236
          shift-left: w238 -> [w244]
          tunnel: w237 -> [w241]
          tunnel: w234 -> [w240] mode=indexing
          tunnel: w232 -> [w239]
          i -> [w242]
          # "Create metadata for\nthe output stream"
          n494 = xnode "Set Dynamic Data Attributes"("Start Timestamp"=w239, "Timestamp"=w241, "Signal Name"=w240, "Signals In"=w244, "Signal Index"=w242) -> ("Signals Out"=w243:dynamicdata)  [unwired: 1 in, 1 out]
        }
        n495 = Enqueue Element(queue=w235, element=w236) -> ()  [unwired: 2 in, 3 out]
      }
    }
    n496 = call "DOut 1"("data"=w168) -> ()  [unwired: 17 in, 2 out]
  }
